vi "ScanDelay_FTIR_BBnorm_Aligning_NewportFlipper_AttenuateBB.vi"() -> ()   [LabVIEW 2022 SP3]
uses:
  Control_scanDelayWorkflow.ctl
  Control_GetSpectrum_BBnorm_AttenuateBB.ctl
panel:
  in  "Norm.smoothing":dbl=1.0 min=0.0 max=100.0 step=0.1
  in  "Flip anyway":bool
  out "Replicated wavelength (nm)":dbl
  in  "Piecewise flattening":i16 min=0 max=10 step=1
  in  "Sample atten.\npowers (%)":dbl[](array[numeric])=[100.0, 75.0, 50.0, 100.0, 100.0, 100.0]
  in  "Sample power (%)":dbl(slide)=100.0 min=0.0 max=100.0 scale=0.0..100.0
  in  "Cyc. per intfg. (BB)":i32=100
  out "Attenuation factor":dbl=1.0
  out "Replication wavelengths":dbl[](array[numeric])=[15000.0, 15000.0, 15000.0, 15000.0, 15000.0, 15000.0, 14286.0, 14286.0, 13333.0, 13333.0, 12500.0, 11765.0, 11111.0, 10526.0, 10000.0, 9524.0, 9091.0, 8696.0, 8333.0, 8000.0, 7692.0, 7407.0, 7143.0, 6897.0, 6667.0, 6452.0, 6250.0, 6061.0, 5882.0, 5714.0, 5556.0, 5405.0, 5263.0, 0.0]
  out "Replicator wavelengths loaded":bool=TRUE
  in  "Replic. path":path=path "C:/Users/mnopl/Desktop/Software/mnOPSuite/PRISM/Alpha replicator tables/2022.10.12_550-2000cm-1_ExtraExtraLowEnergy.txt"
  in  "Load replic. table":bool
  in  "BB attenuation\npowers (%)":dbl[](array[numeric])=[50.0, 1.5, 1.0, 2.0, 2.0, 2.0]
  in  "Attenuation\nenergies (cm-1)":dbl[](array[numeric])=[600.0, 1000.0, 1200.0, 1550.0, 1650.0, 1800.0]
  in  "BB power (%)":dbl(slide)=2.0202020202020203 min=0.0 max=100.0 scale=0.0..100.0
  in  "Power threshold":dbl(slide)=112.33240329780287 scale=10.0..1000.0
  in  "Update alignment":bool
  in  "Bright beam: alignment delay":i32=-11
  in  "Norm phase offset":dbl=14.7
  in  "Bright beam: physical channels (inputV, ScanDelay X)":tag="Dev1/ai2,Dev1/ai3"
  in  "Sample: physical channels (inputV, ScanDelay X)":tag="Dev1/ai6,Dev1/ai3"
  in  "Sample: alignment delay":i32=-2
  in  "Path to save\nnormalized spectrum":path=path "D:/Dropbox/Data/Park-SNOM/2022.10.24 - Alex undeformed STO/STO(Undeformed,S3)-to-Au(S3 x0.25).txt"
  in  "Save normalized\nspectrum":bool
  in  "Optimize\ninterferogram\nalignment":bool
  in  "Toggle BB\nmirror\nUp / Down":bool
  in  "Realign phase":bool=TRUE
  in  "Window FFT":bool=TRUE
  in  "Pause\nacquisition":bool
  in  "Replicate\nfrom #":i8 min=0
  in  "Envelope width":dbl(slide)=2.0303030303030303 scale=0.25..4.0
  out "Accumulated sample BB spectrum":dbl[][](array[numeric])=[[501.8020561554538, 506.7137372169034, 511.62541827835304, 516.5370993398027, 521.4487804012523, 526.3604614627019, 531.2721425241515, 536.1838235856012, 541.0955046470508, 546.0071857085004, 550.91886676995, 555.8305478313996, 560.7422288928493, 565.6539099542989, 570.5655910157485, 575.4772720771981, 580.3889531386478, 585.3006342000974, 590.212315261547, 595.1239963229966, 600.0356773844462, 604.9473584458959, 609.8590395073455, 614.7707205687951, 619.6824016302447, 624.5940826916944, 629.505763753144, 634.4174448145936, 639.3291258760432, 644.2408069374928, 649.1524879989424, 654.0641690603921, 658.9758501218417, 663.8875311832913, 668.799212244741, 673.7108933061907, 678.6225743676403, 683.5342554290899, 688.4459364905395, 693.357617551989, 698.2692986134388, 703.1809796748884, 708.092660736338, 713.0043417977877, 717.9160228592373, 722.8277039206869, 727.7393849821365, 732.6510660435861, 737.5627471050357, 742.4744281664854, 747.386109227935, 752.2977902893846, 757.2094713508343, 762.1211524122839, 767.0328334737335, 771.9445145351831, 776.8561955966327, 781.7678766580823, 786.6795577195319, 791.5912387809816, 796.5029198424312, 801.4146009038809, 806.3262819653305, 811.2379630267801, 816.1496440882297, 821.0613251496793, 825.9730062111289, 830.8846872725785, 835.7963683340282, 840.7080493954778, 845.6197304569275, 850.5314115183771, 855.4430925798267, 860.3547736412763, 865.2664547027259, 870.1781357641755, 875.0898168256251, 880.0014978870748, 884.9131789485244, 889.8248600099741, 894.7365410714237, 899.6482221328733, 904.5599031943229, 909.4715842557725, 914.3832653172221, 919.2949463786717, 924.2066274401215, 929.118308501571, 934.0299895630206, 938.9416706244704, 943.85335168592, 948.7650327473696, 953.6767138088192, 958.5883948702688, 963.5000759317184, 968.4117569931681, 973.3234380546177, 978.2351191160673, 983.146800177517, 988.0584812389666, 992.9701623004162, 997.8818433618658, 1002.7935244233154, 1007.705205484765, 1012.6168865462147, 1017.5285676076643, 1022.4402486691139, 1027.3519297305634, 1032.2636107920132, 1037.1752918534628, 1042.0869729149124, 1046.998653976362, 1051.9103350378116, 1056.8220160992614, 1061.733697160711, 1066.6453782221606, 1071.5570592836102, 1076.4687403450598, 1081.3804214065094, 1086.292102467959, 1091.2037835294086, 1096.1154645908582, 1101.0271456523078, 1105.9388267137574, 1110.850507775207, 1115.7621888366566, 1120.6738698981064, 1125.585550959556, 1130.4972320210056, 1135.4089130824552, 1140.3205941439048, 1145.2322752053547, 1150.1439562668043, 1155.0556373282539, 1159.9673183897035, 1164.878999451153, 1169.7906805126026, 1174.7023615740522, 1179.6140426355018, 1184.5257236969514, 1189.437404758401, 1194.3490858198506, 1199.2607668813002, 1204.1724479427498, 1209.0841290041997, 1213.9958100656493, 1218.9074911270989, 1223.8191721885485, 1228.730853249998, 1233.642534311448, 1238.5542153728975, 1243.465896434347, 1248.3775774957967, 1253.2892585572463, 1258.2009396186959, 1263.1126206801455, 1268.024301741595, 1272.9359828030447, 1277.8476638644943, 1282.7593449259439, 1287.6710259873935, 1292.582707048843, 1297.4943881102927, 1302.4060691717425, 1307.317750233192, 1312.2294312946417, 1317.1411123560913, 1322.0527934175411, 1326.9644744789907, 1331.8761555404403, 1336.78783660189, 1341.6995176633395, 1346.6111987247891, 1351.5228797862387, 1356.4345608476883, 1361.346241909138, 1366.2579229705875, 1371.1696040320371, 1376.0812850934867, 1380.9929661549363, 1385.904647216386, 1390.8163282778357, 1395.7280093392853, 1400.639690400735, 1405.5513714621845, 1410.4630525236341, 1415.374733585084, 1420.2864146465336, 1425.1980957079832, 1430.1097767694328, 1435.0214578308824, 1439.933138892332, 1444.8448199537816, 1449.7565010152312, 1454.6681820766808, 1459.5798631381303, 1464.49154419958, 1469.4032252610295, 1474.3149063224791, 1479.226587383929, 1484.1382684453786, 1489.0499495068282, 1493.9616305682778, 1498.8733116297274, 1503.7849926911772, 1508.6966737526268, 1513.6083548140764, 1518.520035875526, 1523.4317169369756, 1528.3433979984252, 1533.2550790598748, 1538.1667601213244, 1543.078441182774, 1547.9901222442236, 1552.9018033056732, 1557.813484367123, 1562.7251654285726, 1567.6368464900222, 1572.5485275514718, 1577.4602086129214, 1582.371889674371, 1587.2835707358206, 1592.1952517972702, 1597.1069328587198, 1602.0186139201694, 1606.9302949816192, 1611.8419760430688, 1616.7536571045184, 1621.665338165968, 1626.5770192274176, 1631.4887002888672, 1636.4003813503168, 1641.3120624117664, 1646.223743473216, 1651.1354245346658, 1656.0471055961154, 1660.958786657565, 1665.8704677190146, 1670.7821487804642, 1675.6938298419138, 1680.6055109033634, 1685.517191964813, 1690.4288730262626, 1695.3405540877125, 1700.252235149162, 1705.1639162106117, 1710.0755972720613, 1714.9872783335109, 1719.8989593949605, 1724.81064045641, 1729.7223215178597, 1734.6340025793093, 1739.545683640759, 1744.4573647022087, 1749.3690457636583, 1754.2807268251079, 1759.1924078865575, 1764.104088948007, 1769.0157700094567, 1773.9274510709063, 1778.8391321323559, 1783.7508131938057, 1788.6624942552553, 1793.574175316705, 1798.4858563781545, 1803.397537439604, 1808.3092185010537, 1813.2208995625033, 1818.132580623953, 1823.0442616854025, 1827.9559427468523, 1832.867623808302, 1837.7793048697515, 1842.690985931201, 1847.6026669926507, 1852.5143480541003, 1857.42602911555, 1862.3377101769995, 1867.249391238449, 1872.161072299899, 1877.0727533613485, 1881.9844344227981, 1886.8961154842477, 1891.8077965456973, 1896.719477607147, 1901.6311586685965, 1906.5428397300461, 1911.4545207914957, 1916.3662018529456, 1921.2778829143951, 1926.1895639758447, 1931.1012450372943, 1936.012926098744, 1940.9246071601935, 1945.8362882216431, 1950.7479692830927, 1955.6596503445423, 1960.571331405992, 1965.4830124674418, 1970.3946935288914, 1975.306374590341, 1980.2180556517906, 1985.1297367132402, 1990.0414177746898, 1994.9530988361394, 1999.864779897589], [9.05414272477129e-06, 1.146072070056428e-05, 1.3531434917469873e-05, 1.5257339061957748e-05, 1.7079437144261535e-05, 1.8586424060074166e-05, 1.9304052743786562e-05, 1.999383336317147e-05, 2.1561334770228305e-05, 2.2279284302473234e-05, 2.2799783386304058e-05, 2.3335960682250692e-05, 2.3711409589322383e-05, 2.3012041962517163e-05, 2.092371318189444e-05, 1.8247728538339973e-05, 1.6369451359050923e-05, 1.8071206366236603e-05, 2.2128161852382288e-05, 2.6588390553069066e-05, 3.040115189109792e-05, 3.4074633486252515e-05, 3.663854308845291e-05, 3.8686950213374986e-05, 3.998630059395697e-05, 4.036558448352778e-05, 3.9767897466925815e-05, 3.83635045958129e-05, 3.879241420070519e-05, 4.375572948539814e-05, 4.860211083641365e-05, 5.239661368228191e-05, 5.381305658605131e-05, 5.4605335585803846e-05, 5.456928023046857e-05, 5.330826922593081e-05, 5.155650135346775e-05, 4.963808606724598e-05, 4.7300273768685975e-05, 4.4789283821985914e-05, 4.172821833381964e-05, 3.8522819240302246e-05, 3.534413510043003e-05, 3.109825854574018e-05, 2.789151288182236e-05, 2.477637717894916e-05, 2.1665916765090898e-05, 1.8094472804190557e-05, 1.3885132135543352e-05, 1.3855836966766698e-05, 1.9174946576800012e-05, 2.288883487652522e-05, 2.736044057404942e-05, 3.2660182184323965e-05, 3.805551290684421e-05, 4.1634230858486924e-05, 4.359515344804649e-05, 4.417192112484465e-05, 4.350418637820082e-05, 4.159838227870174e-05, 3.863530651558005e-05, 3.689047831293406e-05, 3.564065659373262e-05, 3.4741453422092514e-05, 3.491100256574226e-05, 3.562501222570058e-05, 3.815400212911604e-05, 4.088615936631992e-05, 4.4000391910526505e-05, 4.695543922507996e-05, 4.8434044740882187e-05, 5.061622452333294e-05, 5.4756769204182285e-05, 5.758236758016324e-05, 5.669735052184797e-05, 5.42170352495056e-05, 5.308083060926907e-05, 4.804897607315596e-05, 4.092594837741294e-05, 3.717690682741493e-05, 3.743689734221249e-05, 4.026107820119904e-05, 4.4954407209320324e-05, 4.7937791250041886e-05, 5.0697804141281584e-05, 5.409179272902676e-05, 5.5051425613154196e-05, 5.943098268745728e-05, 6.02792792414743e-05, 6.196699298401036e-05, 6.397471069494848e-05, 6.66199487409774e-05, 7.127680886195002e-05, 7.458691093424846e-05, 7.731337733913675e-05, 7.785117839195202e-05, 7.53822505861062e-05, 7.056970040413338e-05, 6.291131100671327e-05, 5.2941329091929496e-05, 4.392391802194871e-05, 3.963449945856646e-05, 4.1953719475290424e-05, 4.771653614820673e-05, 5.335544843090435e-05, 5.616090792749654e-05, 5.562053151302489e-05, 5.21377627896389e-05, 4.501523397633283e-05, 3.249677831618434e-05, 1.7141861274259747e-05, 1.5912097509484014e-05, 3.462175484396277e-05, 5.7583346557761405e-05, 7.888606886101375e-05, 9.918158620308137e-05, 0.0001155235452915555, 0.0001289014913062019, 0.00013971733824365195, 0.0001470980604228987, 0.00015492802482606013, 0.00016264966498361625, 0.00016940708362537147, 0.00017497322968332827, 0.00018102746470570247, 0.0001870200933101339, 0.0001903175596330271, 0.00018897095803169608, 0.00018550126083230982, 0.00017557385544742657, 0.0001607038012571914, 0.0001367544362581611, 0.00010578345348198371, 8.546921892384217e-05, 9.52720614452018e-05, 0.00013011849973922022, 0.00019168098489810164, 0.00026725317849966666, 0.0003465746427620213, 0.00042891126018012405, 0.0005125761092231905, 0.0006132560660052971, 0.0007934024917234689, 0.001148817600728305, 0.0017821667597155177, 0.002718769896826103, 0.004011495255399954, 0.005669136912491277, 0.0076513168713931235, 0.009982636477995343, 0.012501134269760187, 0.015024090173468677, 0.017527550291906425, 0.019536079280951586, 0.020963553367104662, 0.021737970184997124, 0.021567120315550893, 0.020651465456608627, 0.019327507634875202, 0.017587385259346063, 0.015027071922176814, 0.01172814204759582, 0.008774676653795286, 0.0058183670585716905, 0.003766850285673133, 0.002212783419764623, 0.0012805222286522478, 0.0009088416748197714, 0.0008030169245465611, 0.0007363552520419021, 0.0006601492505867679, 0.0005736996220301791, 0.00046609251899519294, 0.0003437566881312927, 0.00022903562440392688, 0.00012838136651867715, 6.056117939395001e-05, 5.030059625889761e-05, 9.37824759573024e-05, 0.0001365567600822889, 0.00017761940643246386, 0.00020480688388601666, 0.0002213234600721696, 0.00023091740660175332, 0.00023050029871893855, 0.00022282558171466467, 0.00021176685424416765, 0.00020022832886297797, 0.0001912226868460405, 0.00018495657878795033, 0.00017852095629343115, 0.0001715729510544182, 0.0001653927454598181, 0.00015813440587111882, 0.00014740866431915028, 0.00013075370521333123, 0.00011249410778699135, 9.14522961639837e-05, 7.030504947509215e-05, 4.8274400107189045e-05, 3.182127229372215e-05, 2.4193419332374132e-05, 2.7592839368661025e-05, 3.8138419024464994e-05, 4.7411364923720376e-05, 5.453880382281337e-05, 5.900190986884964e-05, 5.939162416780368e-05, 5.836904180156344e-05, 5.7601729757341124e-05, 5.995501366208591e-05, 6.650413636839761e-05, 7.791655511014081e-05, 9.023797696062717e-05, 0.0001015790770096666, 0.00010948200015457708, 0.00011526639888839689, 0.00011795109028559512, 0.00011608954265675919, 0.00011154380593283861, 0.0001044640218107466, 9.618589325302785e-05, 8.897245175579604e-05, 8.297362182561573e-05, 7.733197817718043e-05, 7.221453820714107e-05, 6.798010472825792e-05, 6.209106017009621e-05, 5.582616105465967e-05, 4.889814882305325e-05, 4.308432303836618e-05, 3.81468507684591e-05, 3.504836304277521e-05, 3.3606430234370614e-05, 3.4892670864467355e-05, 3.740416873433292e-05, 4.014239344052927e-05, 4.236918893226478e-05, 4.540812717648292e-05, 4.750654552892193e-05, 4.88451465477639e-05, 4.999628837926609e-05, 5.0693745130209864e-05, 4.965733153995291e-05, 4.7718157132532524e-05, 4.47814947400894e-05, 4.222961881813198e-05, 4.363887345181102e-05, 4.4957856221667463e-05, 4.51818357062012e-05, 4.386171390158789e-05, 4.201732174854946e-05, 4.069355966749328e-05, 4.057027674774872e-05, 3.956998660491812e-05, 3.7473432147203064e-05, 3.470264995956467e-05, 3.080829371952867e-05, 2.5482362826008645e-05, 1.9424338594941943e-05, 1.5159327710234029e-05, 1.2079206222871872e-05, 1.0651298178296682e-05, 1.2330602779842834e-05, 1.4976309843244352e-05, 1.677832393183783e-05, 1.7707514496502166e-05, 1.8518224272784254e-05, 2.0645123455280968e-05, 2.238958039060859e-05, 2.4439615813823628e-05, 2.6411783669056102e-05, 2.9293749268361072e-05, 3.226870700779618e-05, 3.5575707796609386e-05, 3.8953809781552114e-05, 4.235176618092753e-05, 4.514116087133663e-05, 4.6540114190942e-05, 4.606769214915828e-05, 4.491425812718059e-05, 4.383267184081204e-05, 4.511594164863621e-05, 4.841621611549014e-05, 5.084628744927319e-05, 5.1740258164234994e-05, 5.180678588447729e-05, 5.1365569739836615e-05, 5.05500855713967e-05, 4.8324346627633626e-05, 4.368426081651136e-05, 3.9215637554996545e-05, 3.559618337661666e-05, 3.2627452977102426e-05, 2.9761293070238496e-05, 2.7353219897512085e-05, 2.533622978939261e-05, 2.3270055938289895e-05, 2.161392330779274e-05, 2.0154870308401806e-05, 1.9462572929597903e-05, 2.0037053102543743e-05, 2.121962262822815e-05, 2.207763674218256e-05, 2.318570856142014e-05, 2.352550308647713e-05], [0.6806744259585175, 0.6849882092343899, 0.668495848466184, 0.613823660290151, 0.5670256699905454, 0.5445875440523031, 0.546990064137304, 0.5027971094006224, 0.47163747526178623, 0.48842909948987007, 0.5171189634151799, 0.4957475740429013, 0.4888192862937894, 0.4922446845138241, 0.4830547740167819, 0.4523330038331212, 0.43934481192281666, 0.41091648448910995, 0.3701383178282937, 0.2576704200895707, -0.05406794808844366, -2.9309765509939187, -2.9831352822886825, -3.0198247651169337, -3.0713371549259603, -3.114948189689566, -3.1491367580851777, -3.1451705410699007, -3.129289925753888, -3.125575394129504, -3.106096390749937, -3.100847728135735, -3.135358025017434, -3.1838151253039304, -3.2648924033810016, -3.376909723106753, -3.541691857634501, -3.7798495395501477, -4.02201586442248, -4.195031710908829, -4.347412820078549, -4.456887451307068, -4.546803544906954, -4.635519524113365, -4.66545309054276, -4.68530639093207, -4.691936585983891, -4.708317262997989, -4.544956516040903, -4.084744355381776, -3.5889760371687154, -3.236601839820825, -2.9726808507353693, -2.800779807057664, -2.7200603857023293, -2.645324467735087, -2.5994992809400856, -2.5712444774069074, -2.5101737131124016, -2.3835934415958673, -2.2020112502296567, -1.848566034791038, -1.539120582293457, -1.2876672100153965, -1.1712491575884099, -1.1983291631701047, -1.2457471069620216, -1.3567799632556796, -1.4782346677529863, -1.5469386689494908, -1.6102464660586944, -1.6331750864817036, -1.6709023484297494, -1.6881838117255588, -1.5945841111901449, -1.4564987015925728, -1.3313807472150505, -1.021834509760915, -0.6265802400027387, -0.3933956777218133, -0.23455529944051934, -0.116393575522356, -0.06063583465495674, -0.056672229363642176, -0.0707011853554041, -0.06651556862565093, -0.06701995189815028, -0.08519836384250516, -0.1453752673935758, -0.19104373919919887, -0.24310016886619273, -0.2731146058472622, -0.29908174145078853, -0.3459180439848564, -0.38095926307008954, -0.4168769040451293, -0.4411278698630139, -0.4798539476175496, -0.5449944482579601, -0.6581009327727547, -0.8715676027976937, -1.2508736277829517, -1.6971337421250543, -2.0213691446290594, -2.2040449228837145, -2.266631075624979, -2.2641540356125422, -2.2365377454531417, -2.1599287851486655, -2.0463023119591957, -1.6165662075490066, -0.41549872588223785, 0.21706889676303426, 0.34458978885153213, 0.36340627078730087, 0.36919498924122207, 0.3524838424701317, 0.3204822645118805, 0.2957596233332462, 0.28578266456548057, 0.2848106483127703, 0.29956801355058665, 0.3209924016384131, 0.35097351985282144, 0.3893186436017326, 0.423902712704169, 0.44627800290509206, 0.46298635487752854, 0.47871335326365333, 0.4905963210656376, 0.4841124897370323, 0.45541657032287786, 0.3652951332237495, 0.04303936858528297, -0.7536743878984394, -1.3261829974428108, -1.4696028844701314, -1.4586429486007302, -1.3840109453291167, -1.2516588040654963, -1.0573123759968088, -0.7824538427101194, -0.4474818694363703, -0.13589815712052247, 0.08755263607200398, 0.21642632980081397, 0.2862942277725255, 0.3205893750742272, 0.3326444570982469, 0.32938127045895227, 0.31833349636619657, 0.30329049194792596, 0.2829553232250954, 0.26687390368277114, 0.2555619318755968, 0.2505673029245083, 0.25911595629275597, 0.2772754960838983, 0.2973425409459973, 0.3029649582927613, 0.2827761405262055, 0.23732942507677943, 0.20163466037668648, 0.1331497607854461, 0.0379820195901774, -0.13999981345004334, -0.47795745571318854, -0.929010937914907, -1.1994103072581521, -1.2896615783323253, -1.2653352298683456, -1.2098483095719286, -1.1657699548059104, -1.1471930383624103, -1.1281429911558267, -1.1795391975895133, -1.5039067718021788, -2.6936269684786187, -3.0664592616953006, -3.1193851903000795, -3.0854087414640223, -3.0549441336742693, -3.0184550566806156, -2.985441049200191, -2.9511412813394178, -2.918187087297462, -2.8907032121741385, -2.854900914838226, -2.834920748588893, -2.8245153356991257, -2.819751606455825, -2.81602192316084, -2.8152291411993464, -2.829577389185467, -2.8550562214387445, -2.8903925112420272, -2.9264918455310682, -2.9616994840566666, -3.0002506084331704, -2.999118248425433, -2.845589508335458, -1.7373949316942547, -0.6932921798700211, -0.5384382613525608, -0.4995766927485695, -0.514316046620444, -0.5745218661614621, -0.669775445573983, -0.8239144445259048, -1.0346387042374663, -1.2990121854938654, -1.5986247869854187, -1.8472296623316287, -2.021497282413414, -2.1466514781422963, -2.209378153096481, -2.2424589750897685, -2.266648851082515, -2.2799797005398905, -2.309912237678326, -2.345692915641117, -2.384757375923997, -2.4363018382807486, -2.497667099925217, -2.564332792856057, -2.6256948434904293, -2.6694663154440907, -2.6932662176610767, -2.671755748082959, -2.6121329426752458, -2.50396224079028, -2.405377043888912, -2.261188670924277, -1.961869475625591, -1.5078157042629958, -1.0919329006878589, -0.9008797089504061, -0.7780224728162258, -0.7243893273929989, -0.7048124869470134, -0.7013557014828184, -0.7108512635927231, -0.7253035863197828, -0.75849837833151, -0.8028701121530308, -0.8536743084239977, -0.8917074118238381, -0.9071203609288722, -0.9242697845010359, -0.9038786131617589, -0.8639937766237017, -0.8339523553539512, -0.7597506511491052, -0.6887229433663866, -0.6537523468968877, -0.6544456961542199, -0.6418528873431063, -0.6508048799553668, -0.7173890701039488, -0.8823720275302099, -1.234560542288769, -2.5487899960284257, -3.265859158892774, -3.4350535154588333, -3.5483551781026894, -3.613569542051124, -3.7209267603498977, -3.8838812245739764, -4.105786402002394, -4.4040108873667805, -4.694065779254025, -4.93405521235141, -5.132177325063402, -5.324967330883069, -5.4728872622221445, -5.590032554039752, -5.677328649274422, -5.752216276239508, -5.805457545657504, -5.843483612071168, -5.869153092716736, -5.920157198340206, -5.959502513483272, -6.0264303723496795, -6.140367982249792, -6.326400049319197, -6.6048321771131455, -7.029094864507549, -7.572319323971797, -8.001401477157643, -8.185674079242062, -8.311840842830115, -8.424449363726211, -8.502254435462461, -8.533576338364043, -8.580247369363327, -8.583386316082233, -8.587663480138602, -8.609199879121022, -8.632127356897414, -8.59206944725306, -8.502866290557257, -8.413064474235739, -8.331740024107319, -8.268889123446257, -8.255981731146719]]
  out "Accumulated sample spectrum":dbl[][](array[numeric])=[[501.8020561554538, 506.7137372169034, 511.62541827835304, 516.5370993398027, 521.4487804012523, 526.3604614627019, 531.2721425241515, 536.1838235856012, 541.0955046470508, 546.0071857085004, 550.91886676995, 555.8305478313996, 560.7422288928493, 565.6539099542989, 570.5655910157485, 575.4772720771981, 580.3889531386478, 585.3006342000974, 590.212315261547, 595.1239963229966, 600.0356773844462, 604.9473584458959, 609.8590395073455, 614.7707205687951, 619.6824016302447, 624.5940826916944, 629.505763753144, 634.4174448145936, 639.3291258760432, 644.2408069374928, 649.1524879989424, 654.0641690603921, 658.9758501218417, 663.8875311832913, 668.799212244741, 673.7108933061907, 678.6225743676403, 683.5342554290899, 688.4459364905395, 693.357617551989, 698.2692986134388, 703.1809796748884, 708.092660736338, 713.0043417977877, 717.9160228592373, 722.8277039206869, 727.7393849821365, 732.6510660435861, 737.5627471050357, 742.4744281664854, 747.386109227935, 752.2977902893846, 757.2094713508343, 762.1211524122839, 767.0328334737335, 771.9445145351831, 776.8561955966327, 781.7678766580823, 786.6795577195319, 791.5912387809816, 796.5029198424312, 801.4146009038809, 806.3262819653305, 811.2379630267801, 816.1496440882297, 821.0613251496793, 825.9730062111289, 830.8846872725785, 835.7963683340282, 840.7080493954778, 845.6197304569275, 850.5314115183771, 855.4430925798267, 860.3547736412763, 865.2664547027259, 870.1781357641755, 875.0898168256251, 880.0014978870748, 884.9131789485244, 889.8248600099741, 894.7365410714237, 899.6482221328733, 904.5599031943229, 909.4715842557725, 914.3832653172221, 919.2949463786717, 924.2066274401215, 929.118308501571, 934.0299895630206, 938.9416706244704, 943.85335168592, 948.7650327473696, 953.6767138088192, 958.5883948702688, 963.5000759317184, 968.4117569931681, 973.3234380546177, 978.2351191160673, 983.146800177517, 988.0584812389666, 992.9701623004162, 997.8818433618658, 1002.7935244233154, 1007.705205484765, 1012.6168865462147, 1017.5285676076643, 1022.4402486691139, 1027.3519297305634, 1032.2636107920132, 1037.1752918534628, 1042.0869729149124, 1046.998653976362, 1051.9103350378116, 1056.8220160992614, 1061.733697160711, 1066.6453782221606, 1071.5570592836102, 1076.4687403450598, 1081.3804214065094, 1086.292102467959, 1091.2037835294086, 1096.1154645908582, 1101.0271456523078, 1105.9388267137574, 1110.850507775207, 1115.7621888366566, 1120.6738698981064, 1125.585550959556, 1130.4972320210056, 1135.4089130824552, 1140.3205941439048, 1145.2322752053547, 1150.1439562668043, 1155.0556373282539, 1159.9673183897035, 1164.878999451153, 1169.7906805126026, 1174.7023615740522, 1179.6140426355018, 1184.5257236969514, 1189.437404758401, 1194.3490858198506, 1199.2607668813002, 1204.1724479427498, 1209.0841290041997, 1213.9958100656493, 1218.9074911270989, 1223.8191721885485, 1228.730853249998, 1233.642534311448, 1238.5542153728975, 1243.465896434347, 1248.3775774957967, 1253.2892585572463, 1258.2009396186959, 1263.1126206801455, 1268.024301741595, 1272.9359828030447, 1277.8476638644943, 1282.7593449259439, 1287.6710259873935, 1292.582707048843, 1297.4943881102927, 1302.4060691717425, 1307.317750233192, 1312.2294312946417, 1317.1411123560913, 1322.0527934175411, 1326.9644744789907, 1331.8761555404403, 1336.78783660189, 1341.6995176633395, 1346.6111987247891, 1351.5228797862387, 1356.4345608476883, 1361.346241909138, 1366.2579229705875, 1371.1696040320371, 1376.0812850934867, 1380.9929661549363, 1385.904647216386, 1390.8163282778357, 1395.7280093392853, 1400.639690400735, 1405.5513714621845, 1410.4630525236341, 1415.374733585084, 1420.2864146465336, 1425.1980957079832, 1430.1097767694328, 1435.0214578308824, 1439.933138892332, 1444.8448199537816, 1449.7565010152312, 1454.6681820766808, 1459.5798631381303, 1464.49154419958, 1469.4032252610295, 1474.3149063224791, 1479.226587383929, 1484.1382684453786, 1489.0499495068282, 1493.9616305682778, 1498.8733116297274, 1503.7849926911772, 1508.6966737526268, 1513.6083548140764, 1518.520035875526, 1523.4317169369756, 1528.3433979984252, 1533.2550790598748, 1538.1667601213244, 1543.078441182774, 1547.9901222442236, 1552.9018033056732, 1557.813484367123, 1562.7251654285726, 1567.6368464900222, 1572.5485275514718, 1577.4602086129214, 1582.371889674371, 1587.2835707358206, 1592.1952517972702, 1597.1069328587198, 1602.0186139201694, 1606.9302949816192, 1611.8419760430688, 1616.7536571045184, 1621.665338165968, 1626.5770192274176, 1631.4887002888672, 1636.4003813503168, 1641.3120624117664, 1646.223743473216, 1651.1354245346658, 1656.0471055961154, 1660.958786657565, 1665.8704677190146, 1670.7821487804642, 1675.6938298419138, 1680.6055109033634, 1685.517191964813, 1690.4288730262626, 1695.3405540877125, 1700.252235149162, 1705.1639162106117, 1710.0755972720613, 1714.9872783335109, 1719.8989593949605, 1724.81064045641, 1729.7223215178597, 1734.6340025793093, 1739.545683640759, 1744.4573647022087, 1749.3690457636583, 1754.2807268251079, 1759.1924078865575, 1764.104088948007, 1769.0157700094567, 1773.9274510709063, 1778.8391321323559, 1783.7508131938057, 1788.6624942552553, 1793.574175316705, 1798.4858563781545, 1803.397537439604, 1808.3092185010537, 1813.2208995625033, 1818.132580623953, 1823.0442616854025, 1827.9559427468523, 1832.867623808302, 1837.7793048697515, 1842.690985931201, 1847.6026669926507, 1852.5143480541003, 1857.42602911555, 1862.3377101769995, 1867.249391238449, 1872.161072299899, 1877.0727533613485, 1881.9844344227981, 1886.8961154842477, 1891.8077965456973, 1896.719477607147, 1901.6311586685965, 1906.5428397300461, 1911.4545207914957, 1916.3662018529456, 1921.2778829143951, 1926.1895639758447, 1931.1012450372943, 1936.012926098744, 1940.9246071601935, 1945.8362882216431, 1950.7479692830927, 1955.6596503445423, 1960.571331405992, 1965.4830124674418, 1970.3946935288914, 1975.306374590341, 1980.2180556517906, 1985.1297367132402, 1990.0414177746898, 1994.9530988361394, 1999.864779897589], [7.096082360479396e-06, 1.6220386856729275e-05, 1.2223386866077108e-05, 4.282334903322743e-06, 2.1097332179997113e-05, 1.5931965038395668e-05, 1.4783115049740189e-05, 1.064874887303893e-05, 1.5448597881790268e-05, 1.3470240412791832e-05, 1.2958578997869333e-05, 1.5342759416644122e-05, 3.0360154405360435e-06, 7.328117975916059e-06, 1.11069522683048e-05, 1.348424065152223e-05, 1.5966667764614643e-05, 4.256482081007854e-06, 7.698741492917485e-06, 8.865391382740525e-06, 1.8176244058347554e-05, 1.8973154162308674e-05, 1.0912895095445991e-05, 1.325424212557706e-05, 1.084767493023024e-05, 8.18491392927694e-06, 1.0172923454735038e-05, 8.606235895685828e-06, 7.1929677374480615e-06, 6.208684786759582e-06, 1.3033603740988862e-05, 1.729592544754774e-05, 1.1632791731803707e-05, 6.270479610479669e-06, 1.9015952315639412e-05, 1.5877692037602524e-05, 1.424704035985526e-05, 1.3417783494287481e-05, 4.9624588871503026e-06, 7.920464022574053e-06, 7.754802113000556e-06, 1.2212327060122936e-05, 8.192239421572929e-06, 1.1878952892783207e-05, 7.2610520788568465e-06, 1.2441571480584719e-05, 7.0617603301759675e-06, 8.882572928968195e-06, 9.61627100927289e-06, 1.1613496964703238e-05, 1.2974020437570576e-05, 1.2539589787029214e-05, 1.3706075083989123e-05, 1.1166744177971556e-05, 1.09170847990934e-05, 1.396961345036368e-05, 6.148960410007418e-06, 4.117329979906626e-06, 8.251216270028971e-06, 1.4277654679068755e-05, 1.6989586466865932e-05, 9.830933833137905e-06, 2.5365020050501013e-06, 1.2505769826231134e-05, 9.948332249916361e-06, 2.022298421450121e-05, 2.2104870640054155e-05, 1.5351986693574494e-05, 1.6536808333752614e-05, 8.619346205853348e-06, 4.9269921873958635e-06, 7.539082415766658e-06, 1.1265265208212509e-05, 5.3093876408056685e-06, 1.8267496478440106e-05, 8.418129697236088e-06, 1.668977119652175e-05, 1.437691992133319e-05, 1.0733286491980835e-05, 8.030611362074507e-06, 5.290594276412685e-06, 8.325384417407644e-06, 9.164514378310757e-06, 9.132109210043603e-06, 8.92735511203776e-06, 8.642137938522881e-06, 8.43088721396767e-06, 1.5414142206645658e-05, 1.8917345530536863e-05, 1.6807294558207432e-05, 1.5562644438291655e-05, 2.191328348810439e-05, 1.562190993514149e-05, 2.35758717026132e-05, 1.9461969952376293e-05, 2.1239892281209746e-05, 2.551464670387115e-05, 2.121022896753515e-05, 3.1034869497750934e-05, 3.054262223968249e-05, 2.814065303153361e-05, 3.24239667768052e-05, 3.210108331623405e-05, 2.7097569118739543e-05, 1.9549287586006928e-05, 1.920471433777232e-05, 2.085211165385107e-05, 1.9778428616472202e-05, 1.899682396436571e-05, 2.2360867458495652e-05, 1.2903923483678998e-05, 9.716356015491789e-06, 1.1024458431202365e-05, 2.46070382438526e-05, 1.5794963754151342e-05, 2.1988195738978594e-05, 2.2493434485802777e-05, 2.274916971304642e-05, 1.9043714451361174e-05, 3.2455571822991444e-05, 3.9426946712707426e-05, 3.149836580550327e-05, 2.364862770413785e-05, 3.459382392234399e-05, 3.2561050961055636e-05, 2.9750840723544186e-05, 4.532134256484172e-05, 4.442650356547751e-05, 5.3030150646254015e-05, 5.777877288392492e-05, 5.936488175937551e-05, 5.690611765759707e-05, 7.136207722539052e-05, 8.684952921157855e-05, 9.607880565961691e-05, 0.00010397996424653021, 0.00011251166112605888, 0.00011842748610103626, 0.00013925700343623112, 0.00015837228854517795, 0.00018885798104664812, 0.0002357890120263042, 0.0003266366648277566, 0.0004648887026358305, 0.0006663324974086461, 0.0009375934492479617, 0.001289889201388835, 0.0017096453396765817, 0.002195358775923772, 0.002755687667586425, 0.0032971491483591315, 0.003808239568810946, 0.0043694670800612295, 0.004710317324253723, 0.0049607131589019665, 0.005073330983895903, 0.004967087237416828, 0.004769405674776652, 0.00436718318605272, 0.003898901118832271, 0.00326947860920914, 0.0024247164383817844, 0.0015537542497215198, 0.0009721965292059489, 0.0006385748499156821, 0.0003639037640460496, 0.00017783106662409116, 4.7234590752977354e-05, 5.348402396475515e-05, 7.932582168632317e-05, 0.00010868712870559444, 0.00012073088242670934, 0.0001268464298254565, 0.00010751739967993342, 9.802452444909778e-05, 9.109296479305137e-05, 7.798937791952395e-05, 6.4630360392463e-05, 5.1186347717194496e-05, 4.0165022761351634e-05, 4.020839021217865e-05, 3.352705190877265e-05, 3.659022537370472e-05, 3.6047183378015574e-05, 4.402664879467927e-05, 4.173403239711788e-05, 3.7094326533374566e-05, 3.394696617813053e-05, 4.367802757900978e-05, 3.2407369324367004e-05, 3.0888878509555866e-05, 1.796549087525518e-05, 1.6813720693790422e-05, 1.2809437299114951e-05, 1.5125920904250285e-05, 2.179655521601398e-05, 1.4294757256413644e-05, 2.2769359972224953e-05, 2.272077561802974e-05, 1.501029549552028e-05, 1.5224573132860858e-05, 1.1097189981791928e-05, 2.003415699578107e-05, 2.3507740890240143e-05, 1.930736487515885e-05, 3.205176877613794e-05, 3.086052880894781e-05, 3.3237639300179554e-05, 2.8189470341541665e-05, 3.111370999854575e-05, 2.6077334296632935e-05, 2.524932846695447e-05, 2.875277983849729e-05, 2.6310361342494755e-05, 1.87381490192934e-05, 1.861669662325644e-05, 1.7149505464031797e-05, 1.529861533541566e-05, 9.48608645730043e-06, 1.647272876786718e-05, 1.394451953490884e-05, 1.482969749153723e-05, 1.3216652858618266e-05, 7.882712972293426e-06, 6.864781536648055e-06, 4.847759809587256e-06, 5.223428548175379e-06, 8.39573915560291e-06, 8.126667526531172e-06, 7.058328123353561e-06, 7.461150127794082e-06, 8.86426238947459e-06, 1.0946980191083884e-05, 1.324259674572552e-05, 7.971177651892419e-06, 6.664935172352915e-06, 7.032122453049047e-06, 1.2270507074891597e-05, 7.013781342280346e-06, 1.611372777133013e-05, 1.951527239201233e-05, 1.3669726488652514e-05, 8.573566860325885e-06, 7.860704247845982e-06, 9.435319117366857e-06, 1.2611836193932327e-05, 1.126447375953876e-05, 6.02637982793345e-06, 1.545897546346109e-05, 9.287884220712906e-06, 1.1464108097064425e-05, 8.891965582088907e-06, 7.082816008008784e-06, 3.394680172403156e-06, 1.2984101675619772e-05, 1.4964963888138804e-05, 9.448127598473755e-06, 1.2011629818937472e-05, 1.283072967680753e-05, 1.2534603065023814e-05, 7.070989746489091e-06, 1.0179637281450386e-05, 1.0538069586795832e-05, 6.852441095224346e-06, 1.2104186559758078e-05, 1.2538628754685724e-05, 8.284175957360816e-06, 8.650858436875346e-06, 6.750854466426396e-06, 8.432146312558232e-06, 4.507974550206405e-06, 1.0949793060888158e-05, 5.95388678352254e-06, 6.307335969170798e-06, 4.074228192718652e-06, 4.8618155781926654e-06, 1.0512250410263202e-05, 9.499415448978633e-06, 6.276383121874037e-06, 8.169746448445238e-06, 1.2036117271404059e-05, 6.996683099276729e-06, 6.372316970241091e-06, 5.0453959969180045e-06, 6.421931102118251e-06, 1.4015419112640523e-05, 8.548924967471335e-06, 1.088449721112743e-05, 6.692844505840714e-06, 9.780322496321983e-06, 7.83291243722902e-06, 8.35343437412176e-06, 1.3834821163292688e-05, 1.0642471950111049e-05, 1.030219925131364e-05, 7.4303662725959695e-06, 9.261497345916458e-06, 1.0674127331454052e-05, 1.295346646167355e-05, 1.1722741477800632e-05, 8.763110544237398e-06, 1.1406670493965474e-05, 1.2084041085027556e-05, 6.511018285955797e-06, 3.1419452991251818e-06, 6.047792812633947e-06], [-49.58206727087324, -52.06823293132049, -51.59677155767573, -52.31870069711781, -51.991164639108284, -51.05693027011136, -50.388390585021135, -50.67510232822931, -50.148745454930285, -53.19109093769427, -51.59616890898501, -49.96997724661843, -48.0637440852836, -46.17832069695589, -43.88779727601798, -44.54071428292487, -42.719929996739, -40.48253787695988, -38.13418935805937, -37.44789397470244, -36.369339805662136, -34.661575729363946, -32.53811809218756, -29.724037280654372, -27.318578053390738, -26.131113368174013, -25.79138634660744, -24.413830697153386, -24.532049098619993, -21.764139444463908, -19.768588590293476, -16.904423615168056, -15.570603067658666, -13.077056978181318, -11.922224489987983, -12.150316898367223, -10.859554185796085, -9.555622558304847, -7.624387873499771, -7.122390410818255, -7.266142534643009, -8.506066182506473, -6.762533961779596, -7.23859596712073, -8.583196058775755, -9.572516841189682, -8.231903811169232, -9.235464477024479, -9.316455438966969, -9.140920833410874, -9.165660825724288, -9.680412780771334, -9.394099306692553, -7.740358590358383, -7.804716406592078, -8.925910170046748, -7.57252877256316, -6.250146386562463, -8.288095994787668, -11.017446200235447, -9.175535888420548, -7.8714018716313845, -9.33669805879942, -9.349482128480396, -7.579829340238554, -10.48837944093927, -9.243334601881742, -10.27406749916372, -13.373102938096189, -11.771583040025796, -9.21987630645068, -10.457115391902867, -8.549877711788348, -5.588156527718432, -4.656552923516294, -4.352100257965269, -3.8128743676231167, -2.8369355809127157, -3.7777039410185225, -2.5078836341545454, -4.464358062030122, -5.47326755731185, -6.315870510377117, -9.023631774872982, -8.14176682870054, -5.648951000074462, -5.396575095619781, -2.7492283187998083, -0.9476749901979957, -1.6535079167293674, -1.9041012103507313, -1.4642522324003409, -1.5544175568067686, -1.5862247887869927, -1.4188927451235003, -1.3485365725741332, -1.4978984991802946, -1.6074631511796866, -1.1231856063554773, -0.9674954935016871, -0.9818292032517348, -1.4696951158149005, -1.3943436596178884, -1.2797707350272987, -1.0581472172672335, -1.2566924155893986, -0.8188802017241841, -0.934487379800018, -0.9201508576581574, -0.8364985504163798, -0.4854912152201365, -1.4813900102695783, -0.7551172904152708, -0.18569378918256518, 0.07691737929418707, -1.1067773466845523, -1.4570209687139908, -1.4317325333093294, -1.8580990895404312, -1.8836080909858168, -1.8368883765418644, -1.7590184052697708, -1.9554674043154279, -2.234847762600097, -1.7982446396746212, -2.2599299474556886, -2.1052395914099264, -2.022429445515499, -2.2702555833974003, -2.139098256382553, -2.400331377785264, -2.4125836446621207, -2.6703271276350478, -2.566581062856258, -2.7238206966689944, -2.7127621763842598, -2.7730758686688404, -2.9458740203269116, -2.897110094191291, -2.8571493576734355, -2.8373664847177764, -2.789842488116605, -2.7757876198668185, -2.7750969076867165, -2.730127253418047, -2.7416641966174637, -2.7615314886291316, -2.788149687873002, -2.8353974886299653, -2.865116417263593, -2.8976318239663357, -2.9525226237125963, -2.97852944270862, -3.0024743818616884, -3.031683030306553, -3.0314645913611997, -3.027047843178096, -2.9961596717096057, -2.9545397818372265, -2.93792034496191, -2.893638449305101, -2.8121468103189358, -2.9260995910297964, -2.963667938530378, -3.0741187876374028, -3.1249756345830946, -3.208674732285303, -3.597217737260891, -5.483519754354077, -5.849387636033342, -6.107262165211566, -6.140145056889352, -6.252678204666651, -6.250619717512635, -6.488896368472453, -6.44033235404315, -6.630118959397677, -6.635956163171599, -6.645818717841124, -6.528222838020028, -6.782348468449399, -6.708849169444861, -6.696444077887023, -6.746235629551208, -6.869028965930269, -6.861332623423706, -6.8207636106367175, -6.7994720656315195, -6.7998474237918884, -7.029169630898181, -6.992351732359666, -6.777250448594103, -7.012111012549369, -7.687826633074607, -7.437548686596088, -8.063193909697944, -8.340006034282496, -8.716808131153456, -8.439096372686564, -8.147286025639588, -6.9415702894675775, -8.045011049509114, -7.580931436108514, -7.278739704809638, -8.13649827499357, -7.772894666352457, -7.889164155367823, -7.827692780635076, -7.171712771117299, -7.296158022817778, -7.554901035468859, -7.7345530842275, -7.5111826383695615, -7.552248052429306, -7.550781763096708, -7.230642596223063, -7.447324426323249, -7.443610631135627, -7.439725797384867, -7.606296531013399, -7.785323317576015, -7.475011106511161, -6.98167908922936, -7.79089759710682, -6.726106551116871, -8.109015219159133, -7.462237261982594, -4.612723471222822, -3.7935231140733805, -5.216090924702357, -5.248598774188807, -4.15991094699082, -3.725230144267144, -6.858093955335086, -5.139396101609272, -5.360861136852755, -4.82214956875297, -3.753053779923313, -4.7960947914506065, -3.1275337418656264, -2.978161762441438, -2.8095698815112726, -4.079735670874875, -4.713059596127671, -1.7505931592448079, -3.8140547559468203, -3.5360568920327538, -2.2649426038786444, -0.04791412174990484, 0.6294052053287018, 0.1183832889078289, -0.548293474591425, 0.30766352864960567, -1.7009549342943515, -0.550868614347543, -0.387315192474297, -0.13119382138075508, -0.11547347909527872, -0.05089839595212453, -0.28486093981741334, 0.00043449825215446936, 1.0503147223107234, 0.15034553551333119, 1.5821608828076634, 1.899500705696532, -0.9754453882874543, -1.2905127638921385, -3.551211483864641, -6.297299968077951, -5.925915245102473, -8.303942056630753, -5.397154039382862, -8.31777800886968, -8.153461845292213, -5.929076766532205, -4.357415624658813, -1.9649943371332768, -0.6518423485552489, 0.35304915013031746, -2.1529003478899753, -0.2789829941474906, -0.8275960523606543, -1.5990956142781485, -1.2574528112380037, -1.1135107717981256, -1.0064545345404312, -0.6643235747175353, -2.1960638520043503, -1.4188220786783106, -1.68474878666958, -1.2845902439258552, -2.166556808127261, -1.962834740839405, -1.091371297982782, -0.9027447081329498, -1.963763228870782, -1.6989656292995718, -2.0681239676090044, -1.3241655749037804, -1.9706211964647977, -0.8286421870862952, -2.9765368288182827, -1.735695223359997, -0.9204437331073194, -2.2898437042328084, -1.840430591049298]]
  in  "BB-reference spectrum":bool
  in  "Acquire only\nBB 100% curve":bool
  in  "Toggle pause (ms)":dbl=4000.0
  out "BB-referenced spectrum (phase)":T1(graph)
  out "BB-referenced spectrum (amplitude)":T2(graph)
  out "Reference BB spectra":dbl[][](array[numeric])
  out "Reference spectra":dbl[][](array[numeric])
  out "Latest alpha cmd":string="@mir setpump 100.0"
  in  "Replicate\nalpha on\naccumulation":bool=TRUE
  out "# Accumulated":i32=2
  in  "Accumulate to #":i32=2
  in  "Cancel\nacquisition":bool
  out "Toggle position":i32=2
  out "Spectrum stored":bool=TRUE
  out "Reference stored":bool=TRUE
  out "Normalized spectrum (phase)":T1(graph)
  out "Normalized spectrum (amplitude)":T1(graph)
  in  "Store as reference":bool
  out "Python alpha rep path":path=path "C:/Users/mnopl/Desktop/software/mnOPSuite/PRISM/python/alpha.py"
  out "Activity status":string="Awaiting command"
  out "Acquisition status":string="Ready to acquire spectrum"
  in  "Path to save spectrum":path=path "D:/Dropbox/Data/Park-SNOM/2022.10.24 - Alex undeformed STO/Au(S3 x0.25).txt"
  in  "Load reference":bool
  in  "Path to load reference":path=path "D:/Dropbox/Data/Diagnostic/2022.11.02 - PRISM 100% lines/After colinearizing beam path/Au(4).txt"
  in  "Path to load spectrum":path=path "D:/Dropbox/Data/Diagnostic/2022.11.02 - PRISM 100% lines/After colinearizing beam path/Au(3).txt"
  in  "Apply spectral\nenvelope":bool=TRUE
  out "Binned interferogram":cluster{"X":dbl, "Y":dbl}[](graph)
  out "Sample BB Spectra":dbl[][](array[numeric])
  out "Sample Spectra":dbl[][](array[numeric])
  out "Python error: spectrum acquisition":errorcluster
  out "Python scandelay path":path=path "C:/Users/mnopl/Desktop/software/mnOPSuite/PRISM/python/scandelay_FTIR.py"
  in  "Time per\nacquisition (s)":dbl=0.18
  in  "Sampling rate":dbl=250000.0
  in  "Delay calibratior\nfactor (ps/V)":dbl=-2.38 format="%_6g"
  in  "Cyc. / intfg.\n(sample)":i32=100
  out "Accumulated spectrum (amplitude)":T3(graph)
  out "Acquisition cycle":dbl[][](graph)
  out "% averaged":dbl=100.0
  in  "Halt program":bool=TRUE
  out "Python error: activity loop":errorcluster
  in  "Load spectrum":bool
  in  "Save spectrum":bool
  in  "Normalize spectrum":bool
  in  "Acquire spectrum":bool
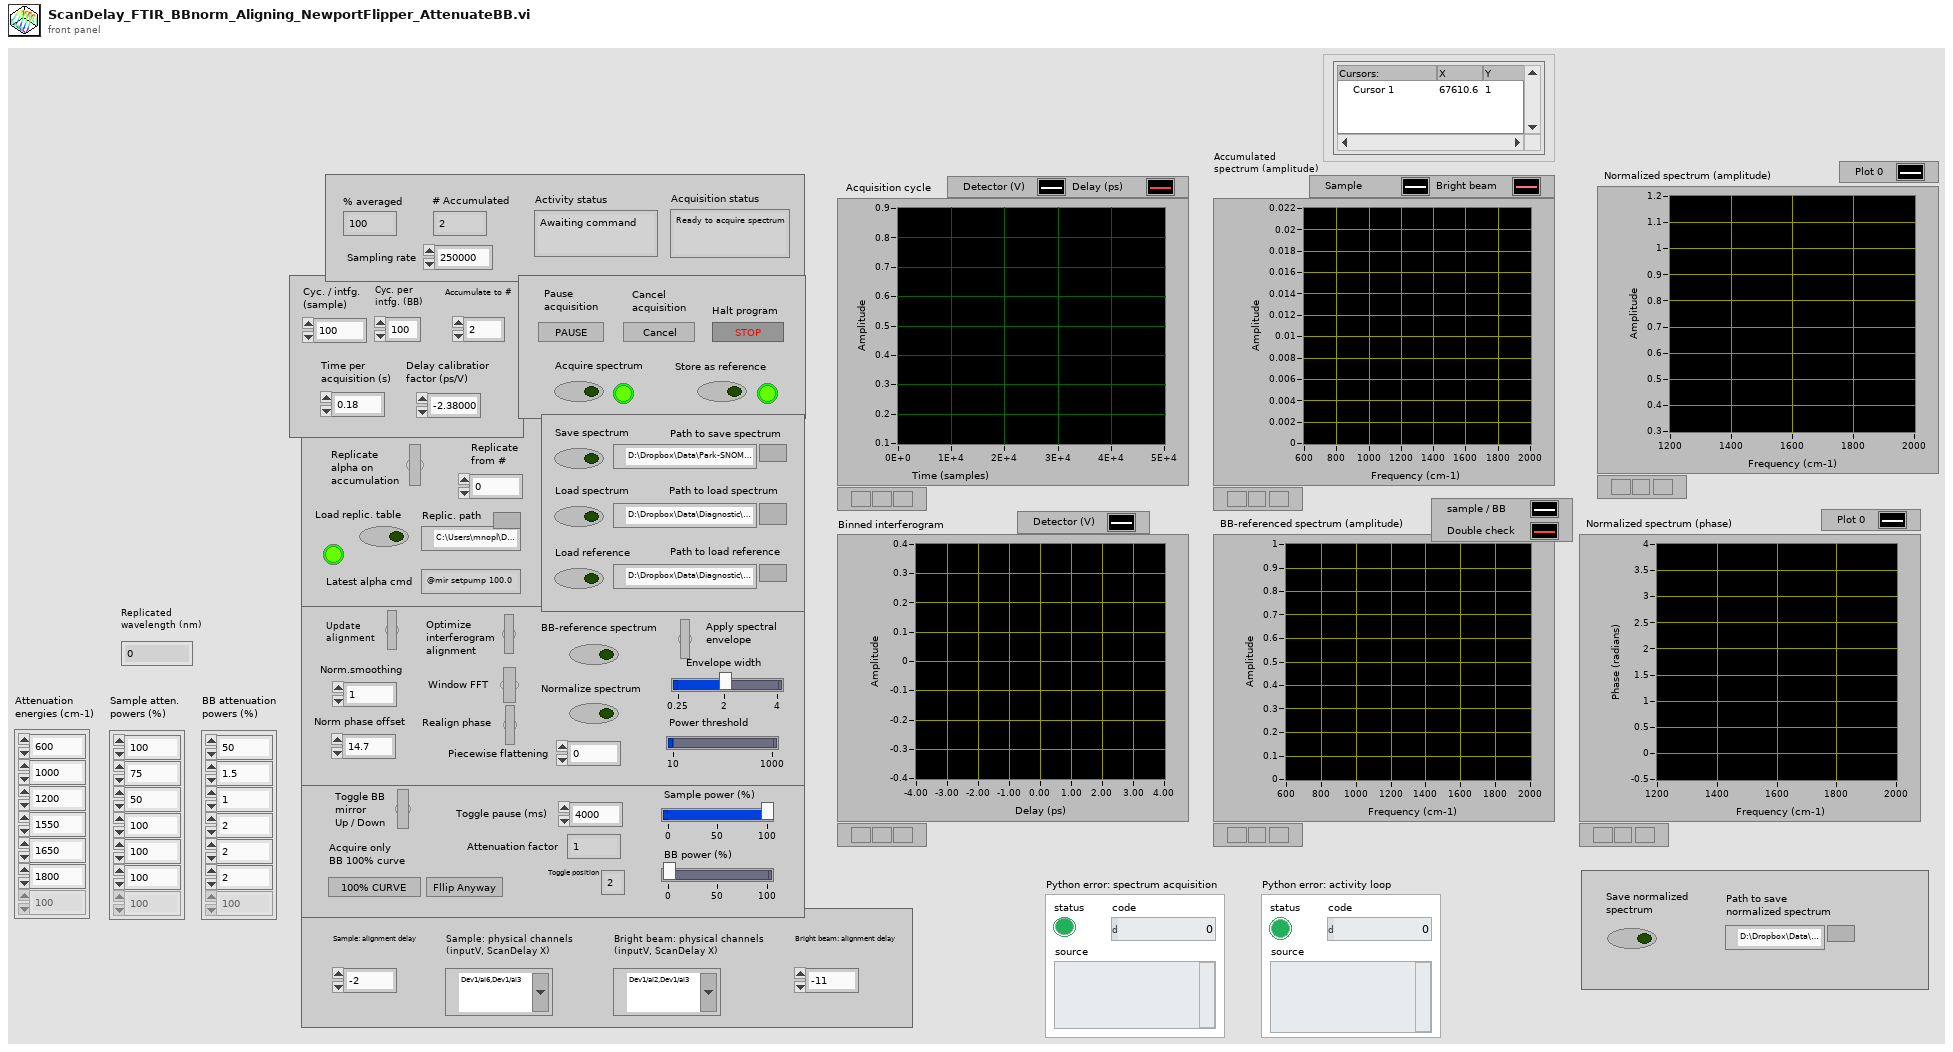
[diagram p1: front panel]
types:
  T1 = cluster{"Output spectrum":dbl[], "Output spectrum":dbl[]}
  T2 = cluster{"Sample Spectra":dbl[], "Sample Spectra":dbl[]}
  T3 = cluster{"Output spectrum":dbl[], "Output spectrum":dbl[]}[]
  T4 = typedef "Control_scanDelayWorkflow.ctl" = enum16{"Initialize", "Sit Idle", "Load replicator table", "Flip BB", "Load Spectrum", "Store reference", "Save Spectrum", "Load reference", "Check Reference", "Check Spectrum", "BB reference spectrum", "Normalize Spectrum", "Save normalized spectrum", "Done"}
  T5 = typedef "imagedata.ctl" = cluster{"image type":i32, "image depth":i32, "image":u8[], "mask":u8[], "colors":u32[], "Rectangle":cluster{"left":i16, "top":i16, "right":i16, "bottom":i16}}
  T6 = typedef "Control_GetSpectrum_BBnorm_AttenuateBB.ctl" = enum16{"Initialize", "Replicate alpha", "Flip in BB", "Attenuate alpha", "Get Spectrum", "Accumulate BB spectrum", "Flip out BB", "Accumulate sample spectrum", "Assess accumulation", "Finalize", "Done"}
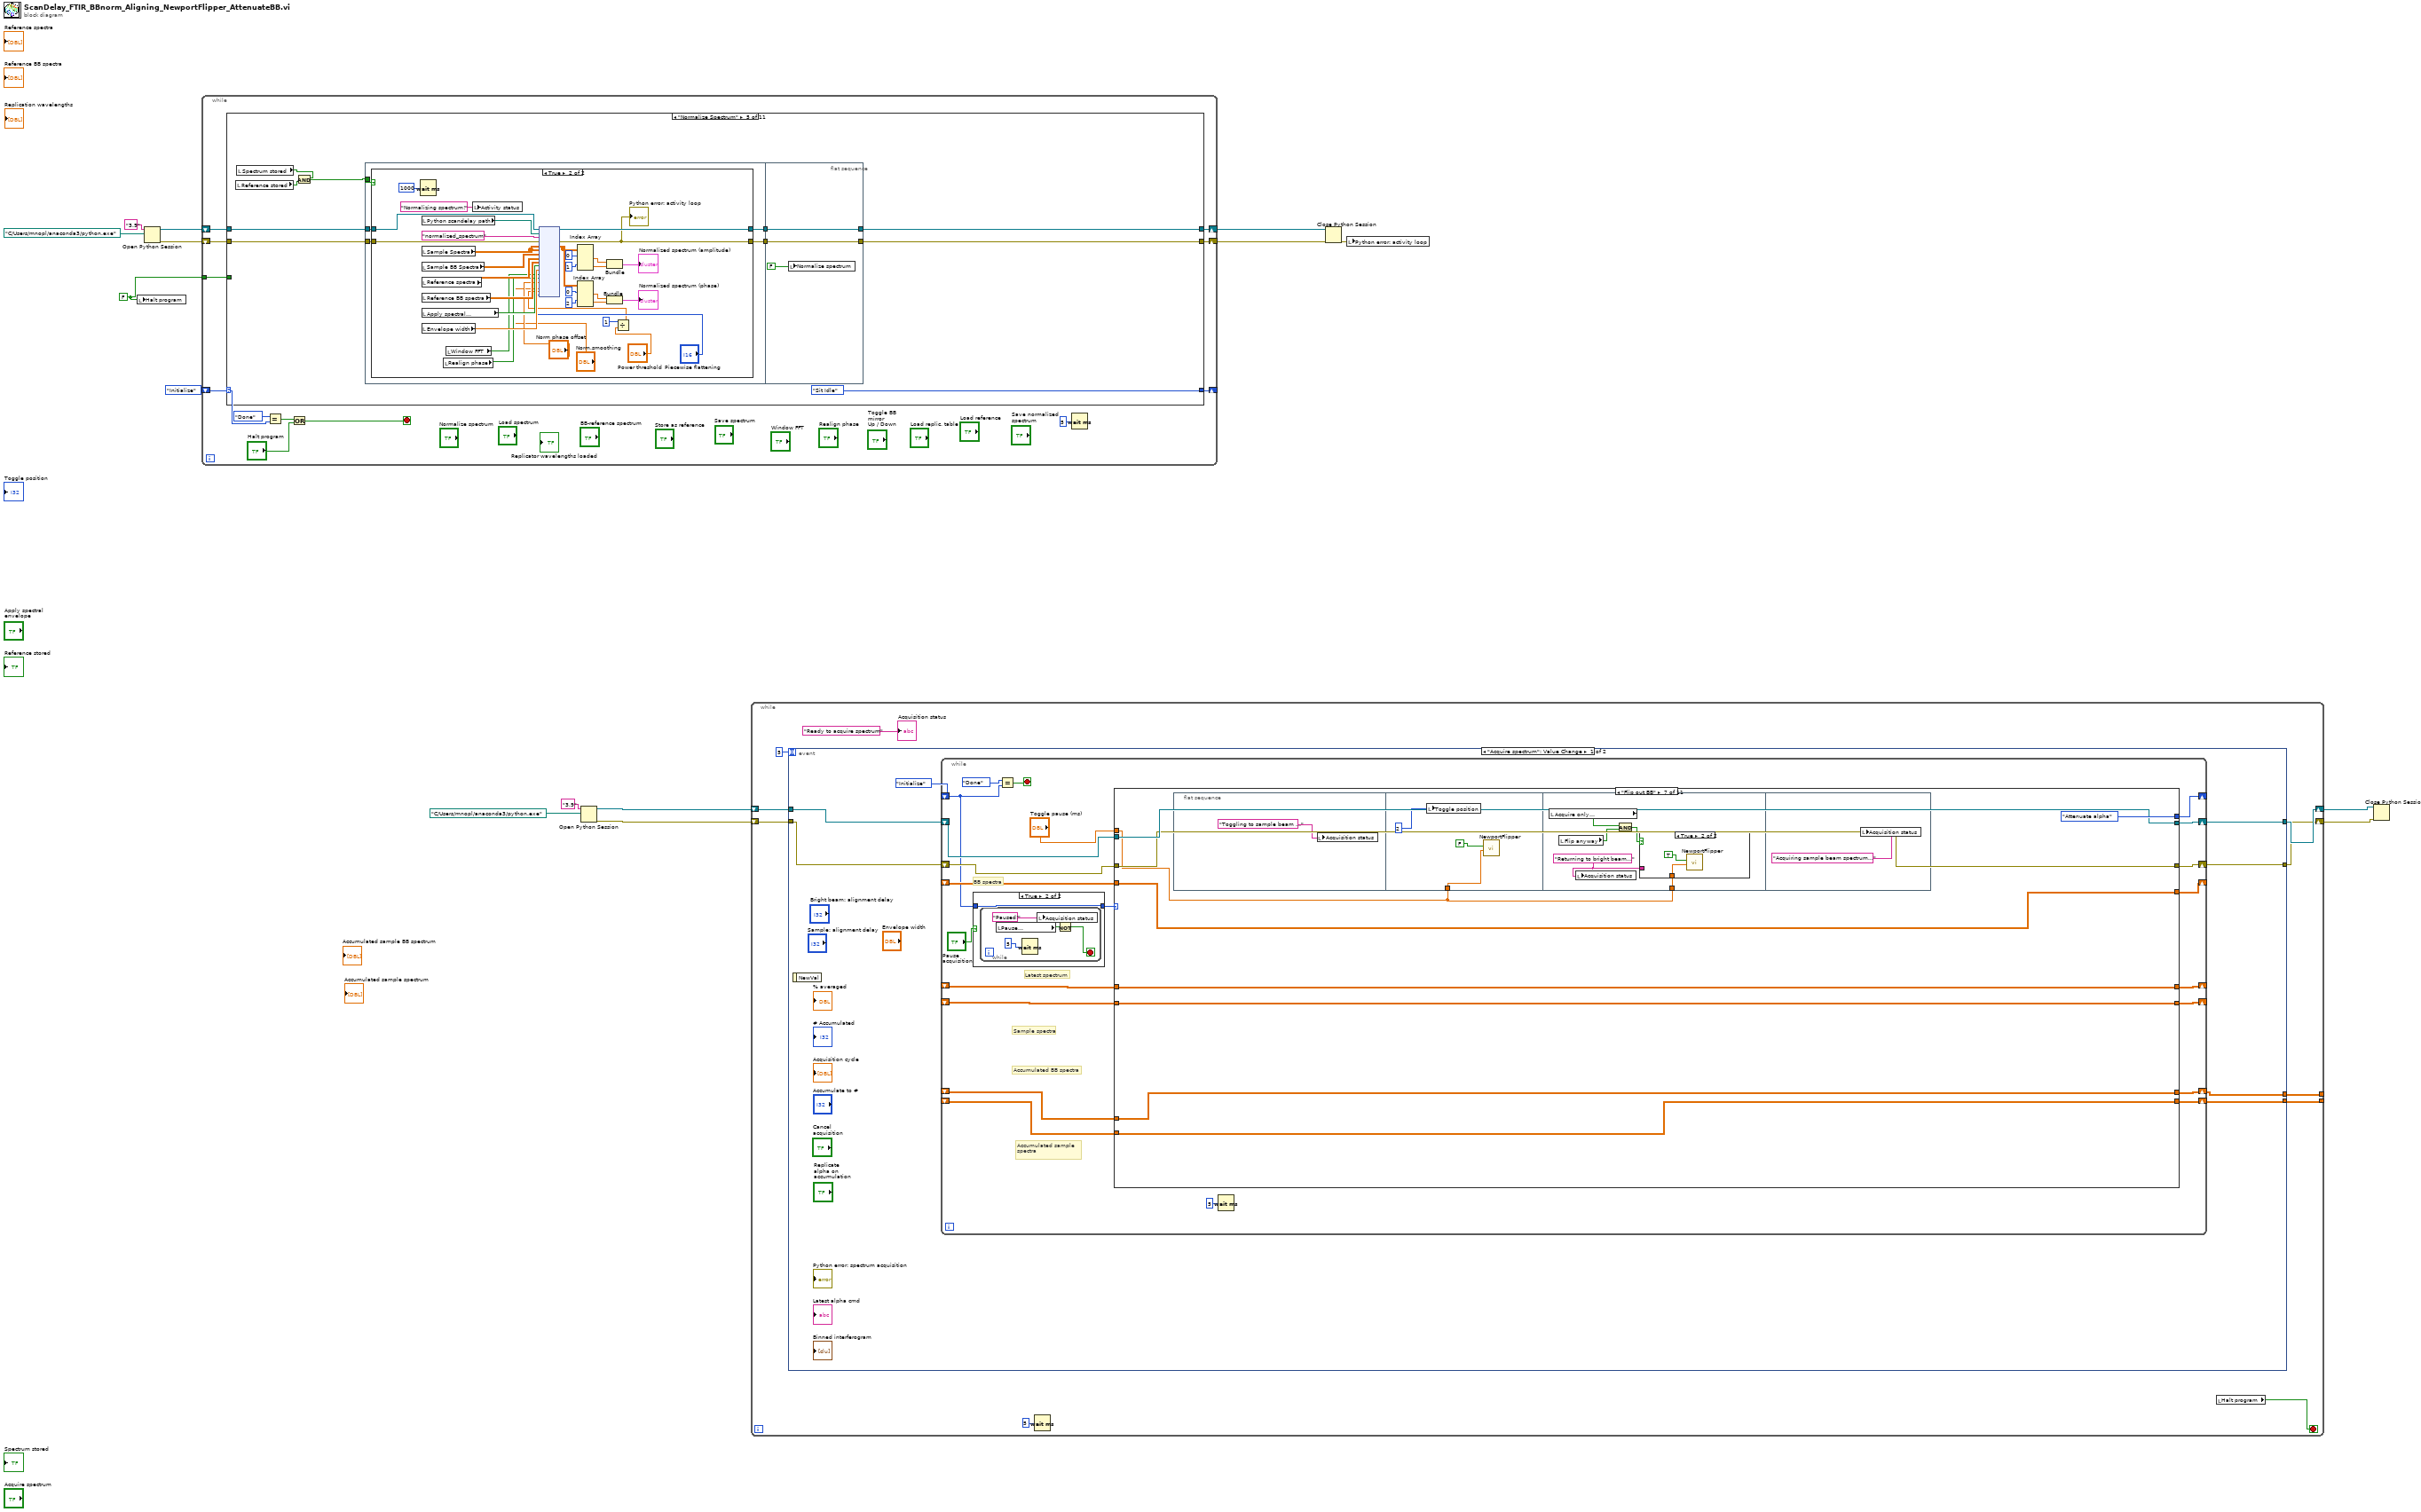
[diagram p0: block diagram]
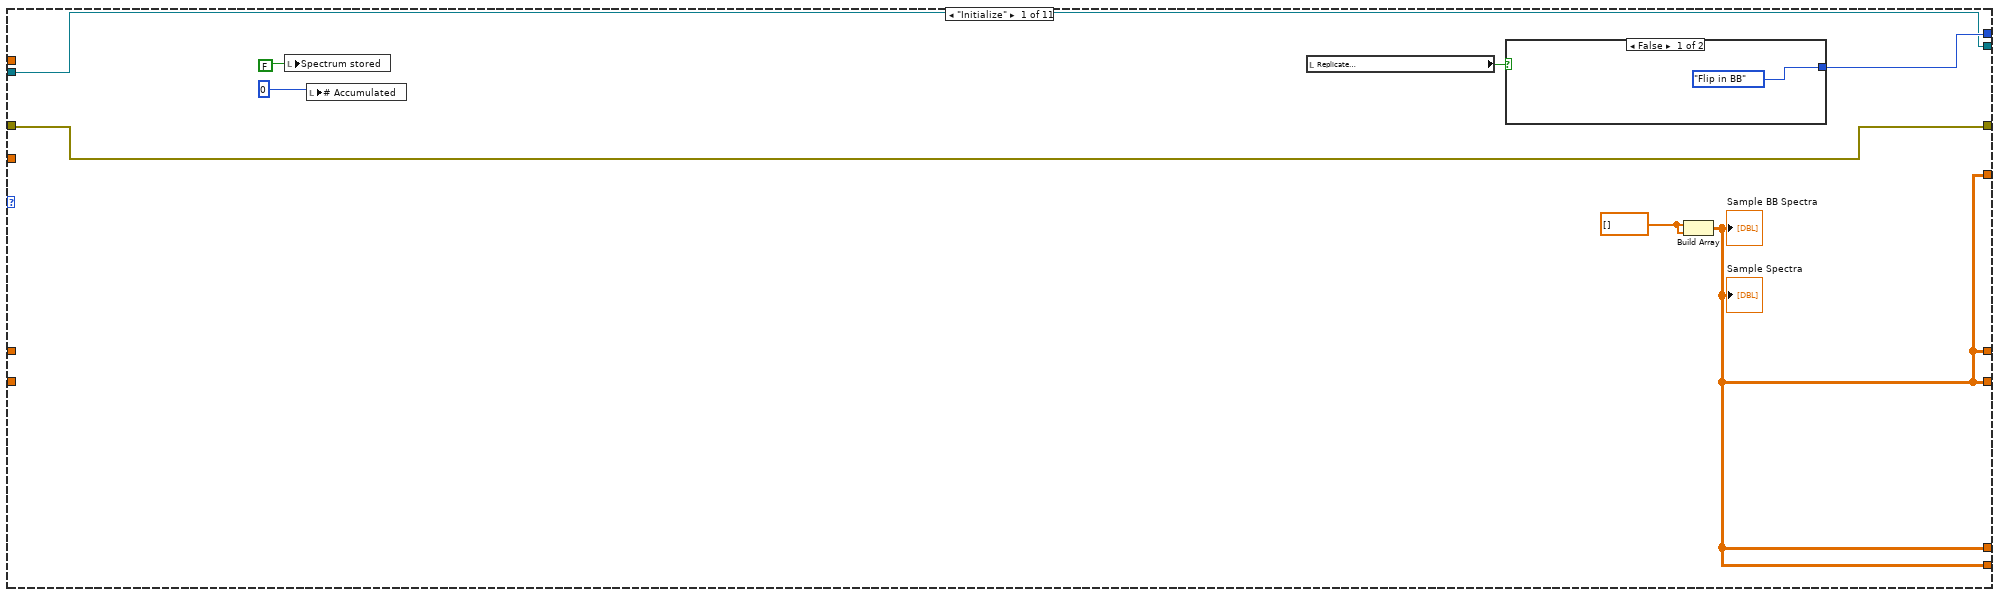
[diagram p3: hidden frame]
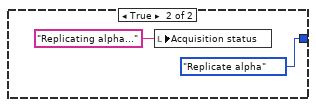
[diagram p4: hidden frame]
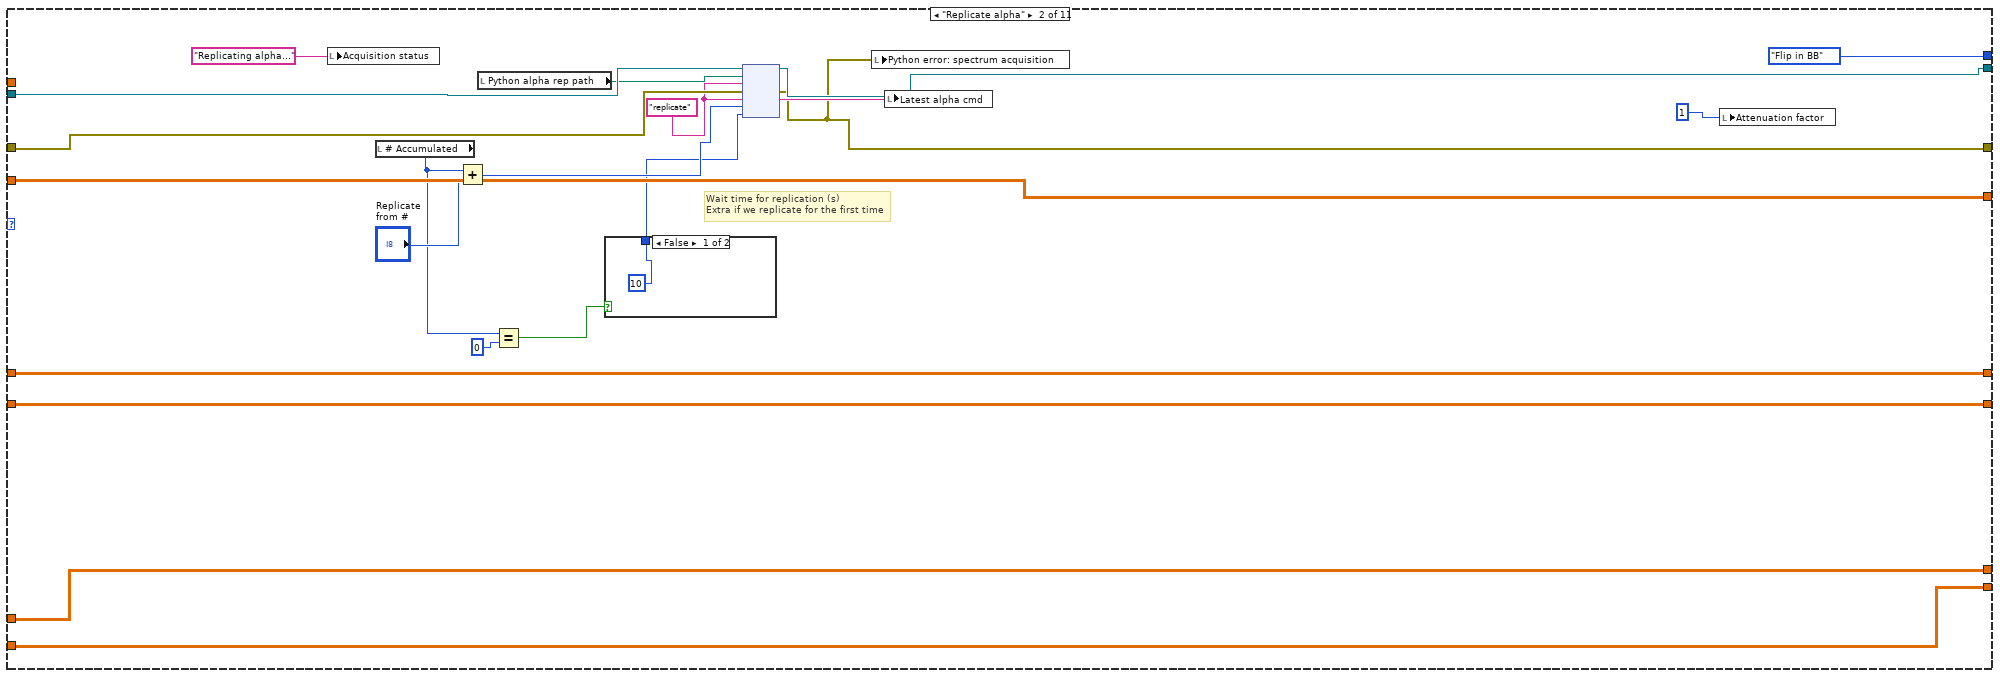
[diagram p5: hidden frame]
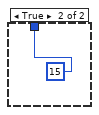
[diagram p6: hidden frame]
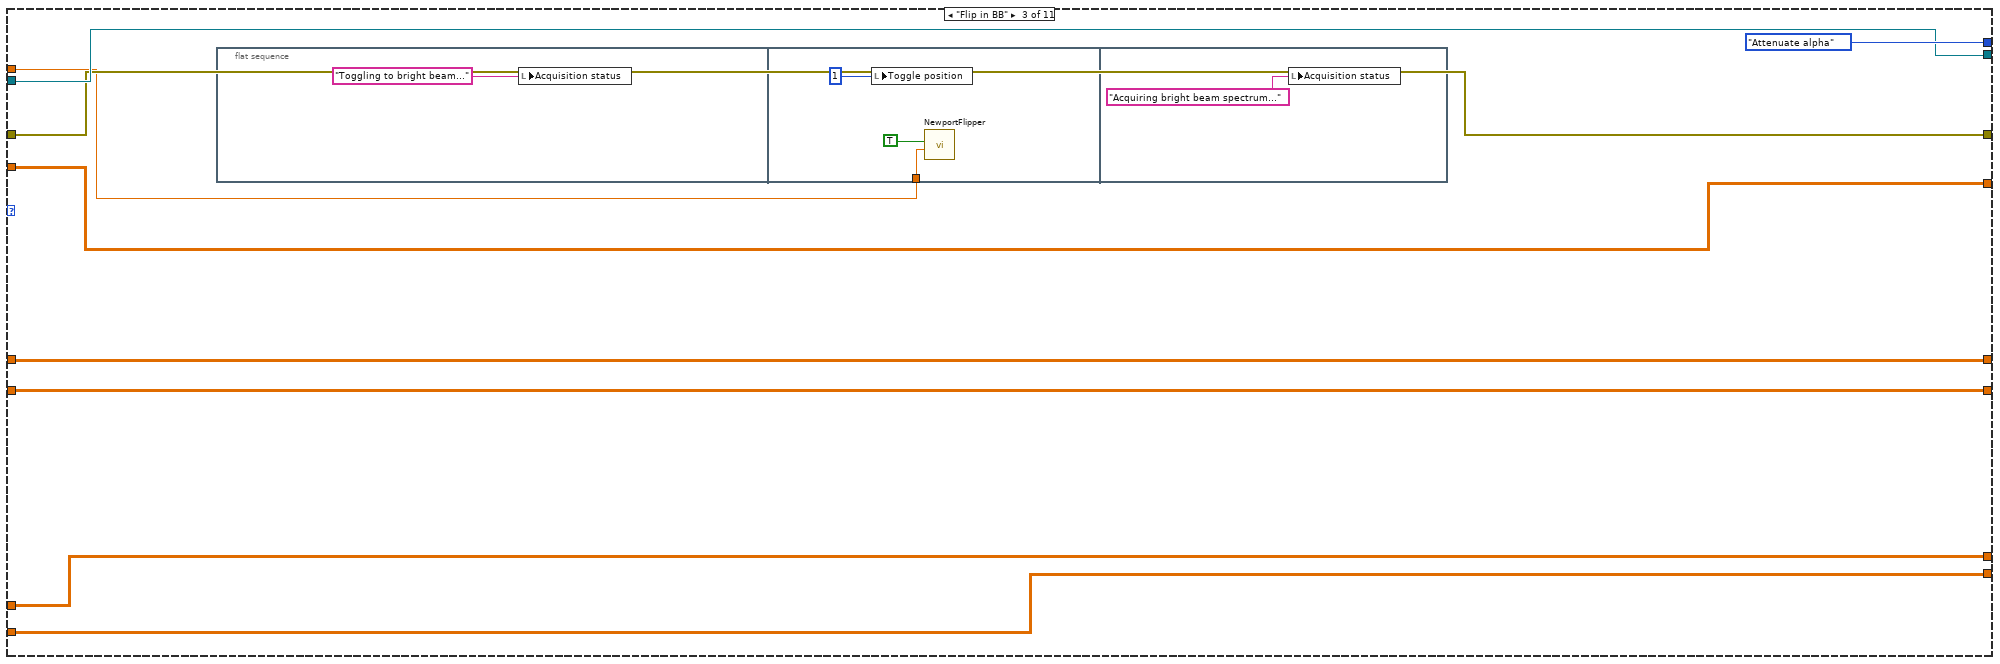
[diagram p7: hidden frame]
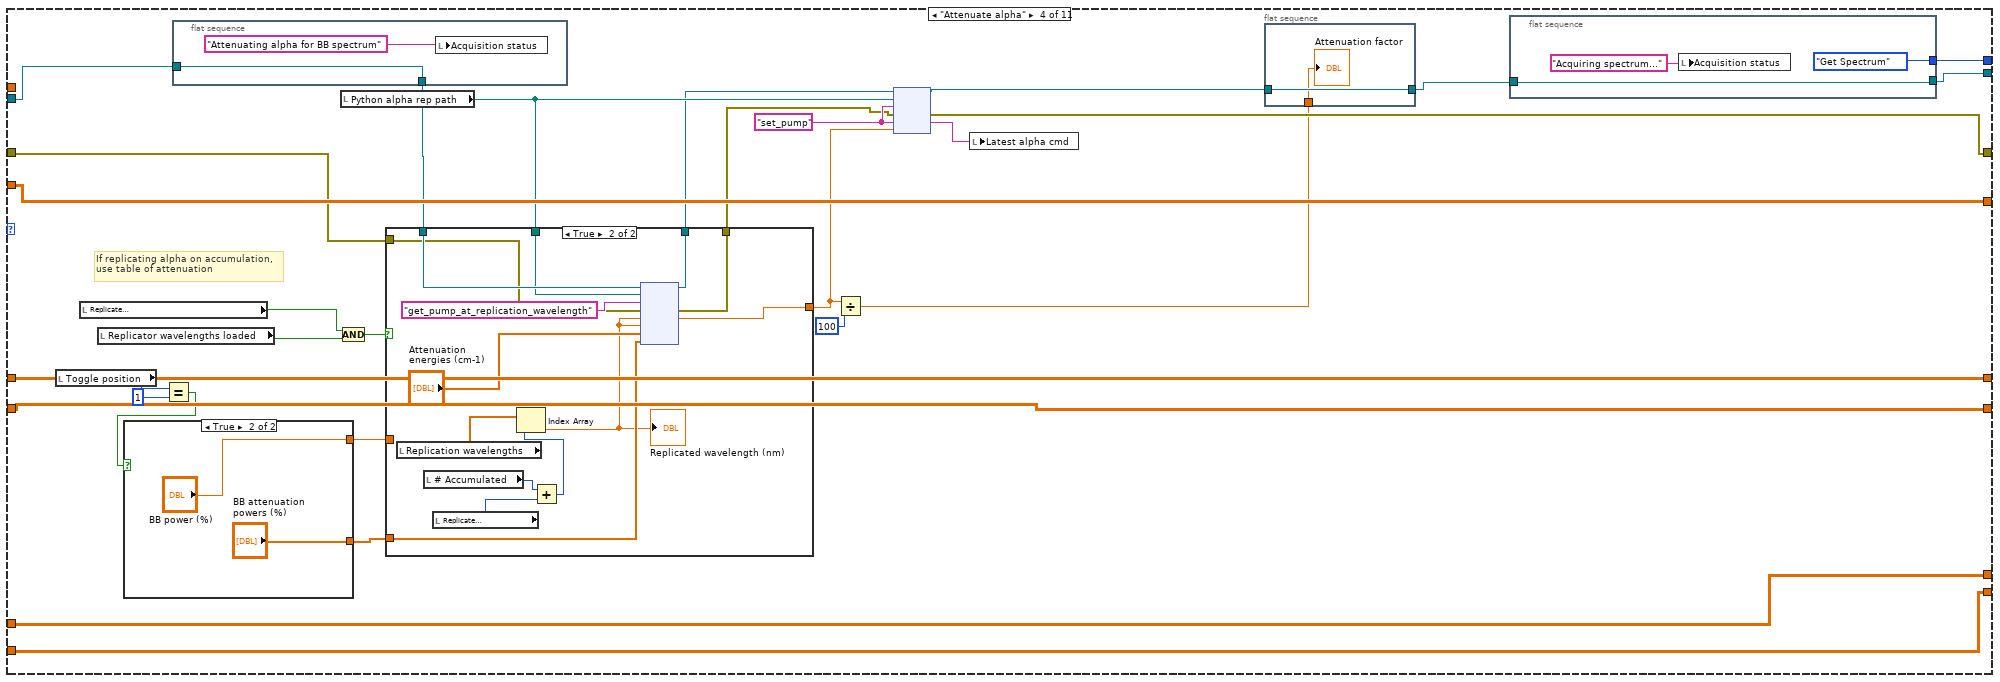
[diagram p8: hidden frame]
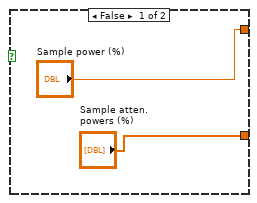
[diagram p9: hidden frame]
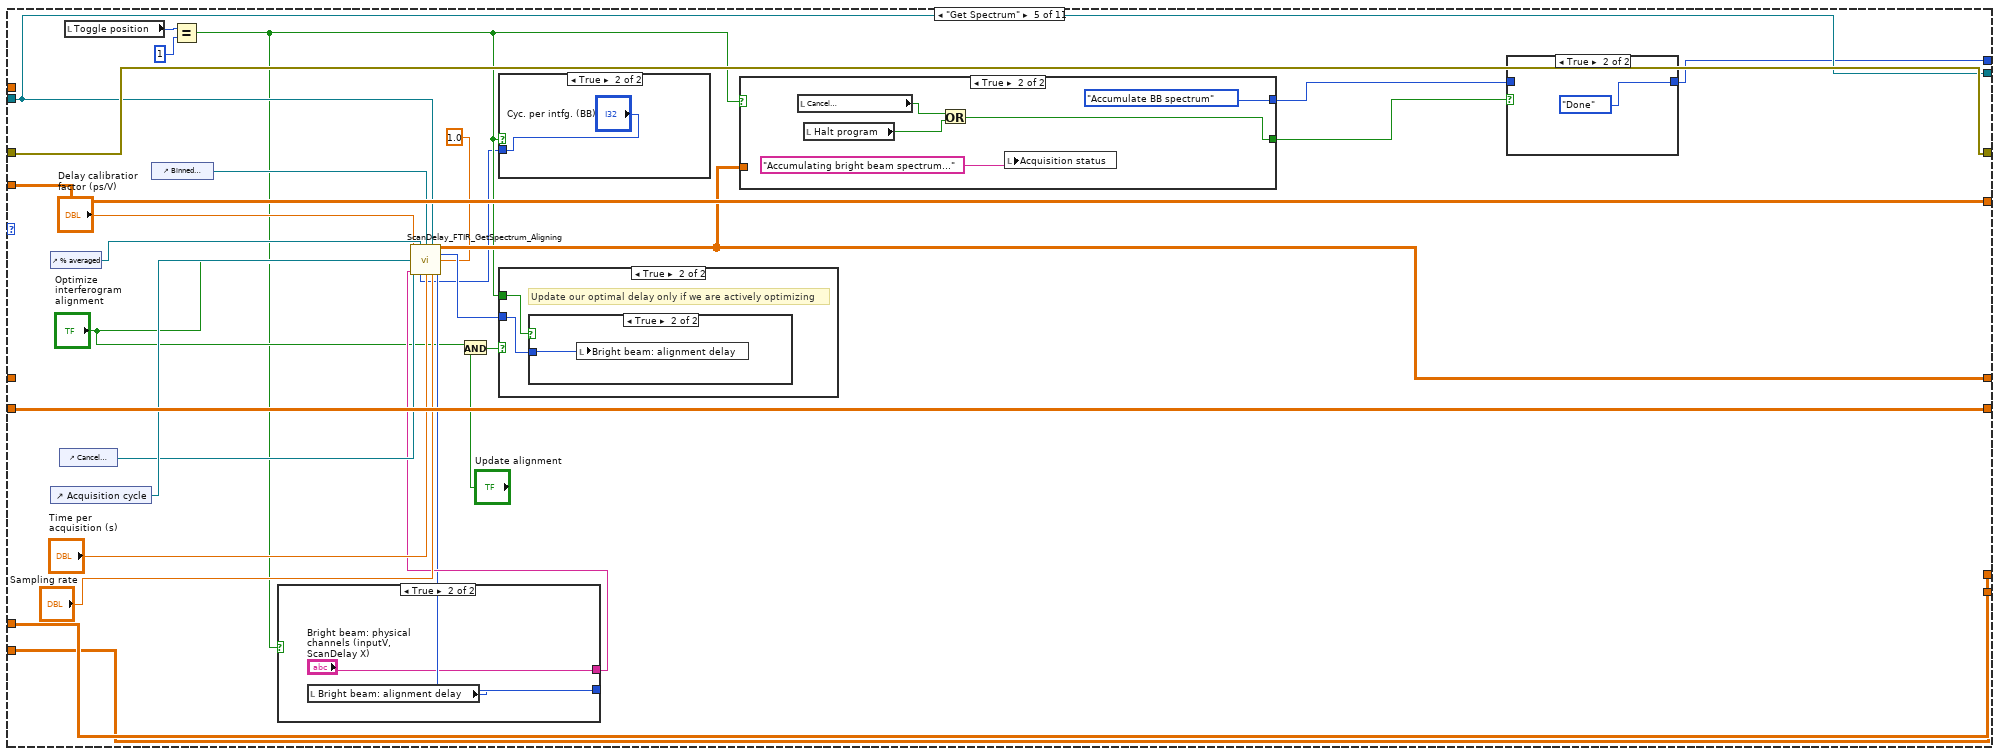
[diagram p11: hidden frame]
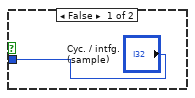
[diagram p12: hidden frame]
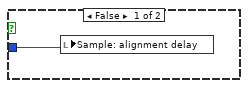
[diagram p14: hidden frame]
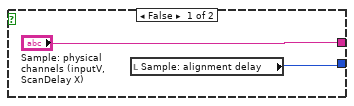
[diagram p15: hidden frame]
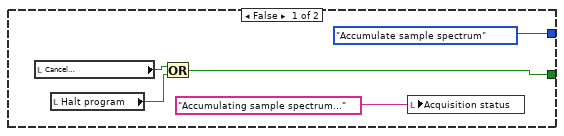
[diagram p17: hidden frame]
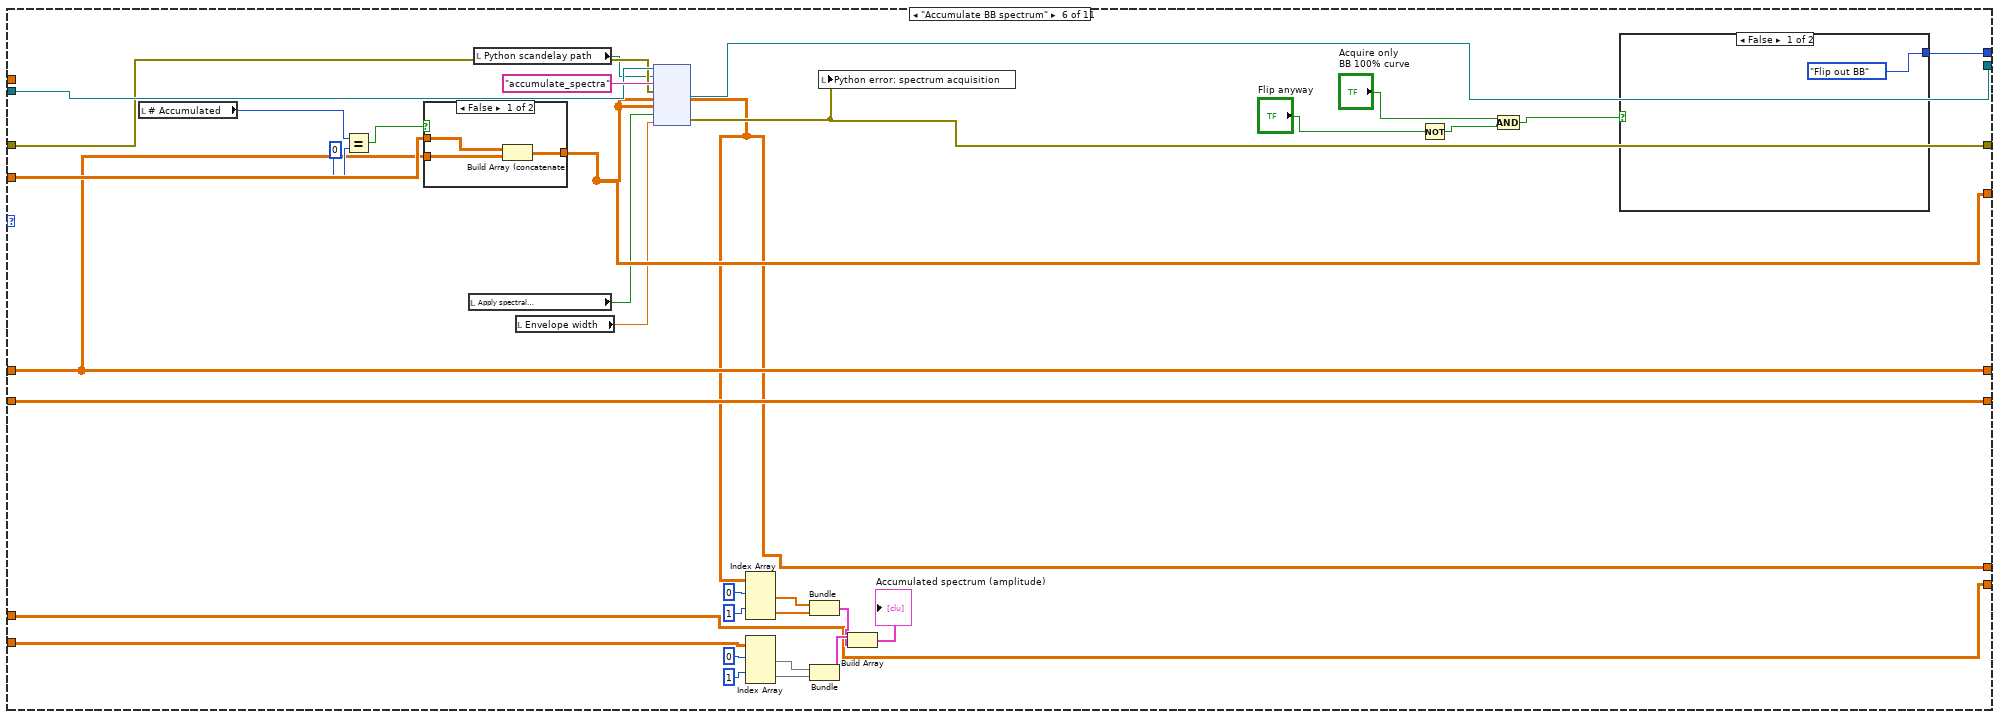
[diagram p18: hidden frame]
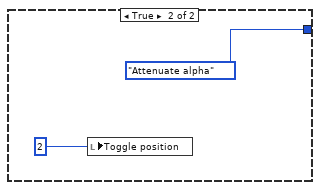
[diagram p19: hidden frame]
diagram:
  w1 = FALSE
  n1 = local write "Halt program"(w1) -> ()
  n2 = Open Python Session(python version="3.9", python path=path "C:/Users/mnopl/anaconda3/python.exe") -> (session out=w11:refnum<k35>, error out=w10:errorcluster)  [unwired: 1 in]
  n3 = while {
    shift-right: [w20] -> _
    shift-left: Control_scanDelayWorkflow."Initialize" -> [w17]
    shift-right: [w26] -> w12
    shift-left: w10 -> [w18]
    shift-right: [w21] -> w13
    shift-left: w11 -> [w19]
    tunnel: w1 -> [w16]
    stop <- w24 stop-if-true
    n4 = case shown="\"Normalize Spectrum\"" w17 {
      tunnel: [w31 w74 w84 w103 w124 w175 w196 w208 w251 w258 w302] -> w26
      tunnel: w19 -> [w32 w73 w83 w104 w127 w176 w197 w206 w252 w259 w303]
      tunnel: w18 -> [w31 w74 w84 w103 w126 w175 w196 w205 w251 w258 w302]
      tunnel: [w32 w73 w83 w104 w125 w176 w197 w207 w252 w259 w303] -> w21
      tunnel: [w30 Control_scanDelayWorkflow."Sit Idle" Control_scanDelayWorkflow."Sit Idle" Control_scanDelayWorkflow."Sit Idle" Control_scanDelayWorkflow."Sit Idle" Control_scanDelayWorkflow."Sit Idle" Control_scanDelayWorkflow."Sit Idle" Control_scanDelayWorkflow."Sit Idle" Control_scanDelayWorkflow."Sit Idle" Control_scanDelayWorkflow."Sit Idle" Control_scanDelayWorkflow."Sit Idle"] -> w20
      tunnel: w16 -> [_ _ _ _ _ _ w193 _ _ _ _]
      frame "Sit Idle", Default {
        n5 = event shown="[5] \"Load replic. table\": Value Change" {
          selector: _ -> [_ _ _ _ _ _ _ _ _ _]
          dyn-events: _ -> [_ _ _ _ _ _ _ _ _ _]
          timeout: 5 -> [_ _ _ _ _ _ _ _ _ w66]
          tunnel: [w33 w37 w44 Control_scanDelayWorkflow."Flip BB" w46 w50 w54 w58 w62 Control_scanDelayWorkflow."Sit Idle"] -> w30
          event "Normalize spectrum": Value Change {
            n6 = event-data() -> ("NewVal"=w34:bool)  [unwired: 1 in]
            n7 = Select(t=Control_scanDelayWorkflow."Normalize Spectrum", s=w34, f=Control_scanDelayWorkflow."Sit Idle") -> (s? t:f=w33:T4)
          }
          event "Store as reference": Value Change {
            n8 = event-data() -> ("NewVal"=w40:bool)  [unwired: 1 in]
            n9 = Select(t=Control_scanDelayWorkflow."Store reference", s=w40, f=Control_scanDelayWorkflow."Sit Idle") -> (s? t:f=w37:T4)
          }
          event "BB-reference spectrum": Value Change {
            n10 = event-data() -> ("NewVal"=w42:bool)  [unwired: 1 in]
            n11 = Select(t=Control_scanDelayWorkflow."BB reference spectrum", s=w42, f=Control_scanDelayWorkflow."Sit Idle") -> (s? t:f=w44:T4)
          }
          event "Toggle BB\nmirror\nUp / Down": Value Change {
            n12 = event-data() -> ()  [unwired: 1 in, 1 out]
          }
          event "Save normalized\nspectrum": Value Change {
            n13 = event-data() -> ("NewVal"=w47:bool)  [unwired: 1 in]
            n14 = Select(t=Control_scanDelayWorkflow."Save normalized spectrum", s=w47, f=Control_scanDelayWorkflow."Sit Idle") -> (s? t:f=w46:T4)
          }
          event "Load replic. table": Value Change {
            n15 = event-data() -> ("NewVal"=w53:bool)  [unwired: 1 in]
            n16 = Select(t=Control_scanDelayWorkflow."Load replicator table", s=w53, f=Control_scanDelayWorkflow."Sit Idle") -> (s? t:f=w50:T4)
          }
          event "Save spectrum": Value Change {
            n17 = event-data() -> ("NewVal"=w55:bool)  [unwired: 1 in]
            n18 = Select(t=Control_scanDelayWorkflow."Save Spectrum", s=w55, f=Control_scanDelayWorkflow."Sit Idle") -> (s? t:f=w54:T4)
          }
          event "Load reference": Value Change {
            n19 = event-data() -> ("NewVal"=w61:bool)  [unwired: 1 in]
            n20 = Select(t=Control_scanDelayWorkflow."Load reference", s=w61, f=Control_scanDelayWorkflow."Sit Idle") -> (s? t:f=w58:T4)
          }
          event "Load spectrum": Value Change {
            n21 = event-data() -> ("NewVal"=w63:bool)  [unwired: 1 in]
            n22 = Select(t=Control_scanDelayWorkflow."Load Spectrum", s=w63, f=Control_scanDelayWorkflow."Sit Idle") -> (s? t:f=w62:T4)
          }
          event Timeout {
            n23 = event-data() -> ()  [unwired: 1 in, 2 out]
            n24 = Wait (ms)(milliseconds to wait=w66) -> ()  [unwired: 1 out]
          }
        }
        "Activity status" <- "Awaiting command"
      }
      frame "Store reference" {
        # "Is spectrum a full array?"
        n25 = local read "Sample Spectra"() -> (w69:dbl[][])
        n26 = local read "Sample BB Spectra"() -> (w68:dbl[][])
        n27 = Empty Array?(array=w69) -> (empty?=w71:bool)
        n28 = Not(x=w71) -> (.not. x?=w70:bool)
        n29 = case shown="True" w70 {
          tunnel: w69 -> [_ w77]
          tunnel: w68 -> [_ w78]
          frame False {
            n30 = Wait (ms)(milliseconds to wait=1000) -> ()  [unwired: 1 out]
            n31 = local write "Activity status"("Error: Spectrum is empty!") -> ()
          }
          frame True {
            n32 = local write "Reference BB spectra"(w78) -> ()
            n33 = local write "Reference spectra"(w77) -> ()
            n34 = local write "Reference stored"(TRUE) -> ()
            n35 = Wait (ms)(milliseconds to wait=1000) -> ()  [unwired: 1 out]
            n36 = local write "Activity status"("Storing reference!") -> ()
          }
        }
      }
      frame "Save Spectrum" {
        n37 = flat-sequence {
          frame #0 {
            w90 = "%g"
            n38 = local read "Sample Spectra"() -> (w92:dbl[][])
            n39 = Path To String(path="Path to save spectrum") -> (string=w94:string)
            n40 = local read "Sample BB Spectra"() -> (w85:dbl[][])
            n41 = Search and Replace String(input string=w94, search string="(.txt)*$", replace string=".txt") -> (result string=w98:string)  [unwired: 5 in, 3 out]
            n42 = Search and Replace String(input string=w98, search string=".txt$", replace string="_BB.txt") -> (result string=w97:string)  [unwired: 5 in, 3 out]
            n43 = String To Path(string=w98) -> (path=w95:path)
            n44 = Array To Spreadsheet String(array=w92, 3:w90) -> (spreadsheet string=w91:string)  [unwired: 1 in]
            n45 = Array To Spreadsheet String(array=w85, 3:w90) -> (spreadsheet string=w99:string)  [unwired: 1 in]
            n46 = String To Path(string=w97) -> (path=w96:path)
            n47 = Write to Text File(file (use dialog)=w95, text=w91) -> ()  [unwired: 2 in, 3 out]
            n48 = Write to Text File(file (use dialog)=w96, text=w99) -> ()  [unwired: 2 in, 3 out]
          }
          frame #1 {
            n49 = local write "Activity status"("Successfully saved spectrum!") -> ()
            n50 = Wait (ms)(milliseconds to wait=1000) -> ()  [unwired: 1 out]
          }
        }
      }
      frame "Load reference" {
        n51 = flat-sequence {
          frame #0 {
            w109 = "%g"
            n52 = Path To String(path="Path to load reference") -> (string=w105:string)
            n53 = Search and Replace String(input string=w105, search string=".txt$", replace string="_BB.txt") -> (result string=w107:string)  [unwired: 5 in, 3 out]
            n54 = Read from Text File(file (use dialog)="Path to load reference") -> (text=w110:string)  [unwired: 3 in, 3 out]
            n55 = String To Path(string=w107) -> (path=w114:path)
            n56 = Spreadsheet String To Array(format string=w109, spreadsheet string=w110) -> (array=w111:dbl[][])  [unwired: 2 in]
            n57 = Read from Text File(file (use dialog)=w114) -> (text=w113:string)  [unwired: 3 in, 3 out]
            n58 = local write "Reference spectra"(w111) -> ()
            n59 = Spreadsheet String To Array(format string=w109, spreadsheet string=w113) -> (array=w115:dbl[][])  [unwired: 2 in]
            n60 = local write "Reference BB spectra"(w115) -> ()
          }
          frame #1 {
            n61 = local write "Reference stored"(TRUE) -> ()
            n62 = Wait (ms)(milliseconds to wait=1000) -> ()  [unwired: 1 out]
            n63 = local write "Activity status"("Successfully loaded reference!") -> ()
          }
        }
      }
      frame "Normalize Spectrum" {
        n64 = local read "Reference stored"() -> (w121:bool)
        n65 = local read "Spectrum stored"() -> (w120:bool)
        n66 = And(x=w120, y=w121) -> (x .and. y?=w119:bool)
        n67 = flat-sequence {
          tunnel: w127 -> [w133]
          tunnel: w126 -> [w132]
          tunnel: [w131] -> w123
          tunnel: [w130] -> w122
          tunnel: w119 -> [w129]
          tunnel: [w172] -> w124
          tunnel: [w173] -> w125
          tunnel: w123 -> [w173]
          tunnel: w122 -> [w172]
          frame #0 {
            n68 = case shown="True" w129 {
              tunnel: w133 -> [w135 w169]
              tunnel: w132 -> [w134 w168]
              tunnel: [w135 w167] -> w131
              tunnel: [w134 w150] -> w130
              frame False {
                n69 = Wait (ms)(milliseconds to wait=1000) -> ()  [unwired: 1 out]
                n70 = local write "Activity status"("Error: Spectrum or reference is empty!") -> ()
              }
              frame True {
                n71 = Wait (ms)(milliseconds to wait=1000) -> ()  [unwired: 1 out]
                n72 = local read "Python scandelay path"() -> (w166:path)
                n73 = local read "Sample Spectra"() -> (w151:dbl[][])
                n74 = local read "Sample BB Spectra"() -> (w152:dbl[][])
                n75 = local read "Reference spectra"() -> (w149:dbl[][])
                n76 = local read "Reference BB spectra"() -> (w148:dbl[][])
                n77 = local read "Apply spectral\nenvelope"() -> (w147:bool)
                n78 = local read "Envelope width"() -> (w146:dbl)
                n79 = local read "Realign phase"() -> (w144:bool)
                n80 = local read "Window FFT"() -> (w145:bool)
                n81 = local write "Activity status"("Normalizing spectrum!") -> ()
                n82 = Divide(x=1, y="Power threshold") -> (x/y=w139:dbl)
                n83 = node(w169, w166, "normalized_spectrum", w168, w151, w151, w152, w149, w148, w147, w146, w145, w144, "Norm phase offset", "Norm.smoothing", w139, "Piecewise flattening") -> (w167:refnum<k35>, w150:errorcluster, w154:dbl[][])  [unwired: 12 in, 2 out]
                "Python error: activity loop" <- w150
                n84 = Index Array(array=w154, index (row) #1=0, index (row) #2=1) -> (element #1=w162:dbl[], element #2=w161:dbl[])  [unwired: 2 in]
                n85 = Index Array(array=w154, index (row) #1=0, index (row) #2=2) -> (element #1=w158:dbl[], element #2=w157:dbl[])  [unwired: 2 in]
                n86 = Bundle("Sample Spectra"=w162, "Sample Spectra"=w161) -> (→"Normalized spectrum (amplitude)":T2)  [unwired: 1 in]
                n87 = Bundle("Sample Spectra"=w158, "Sample Spectra"=w157) -> (→"Normalized spectrum (phase)":T2)  [unwired: 1 in]
              }
            }
          }
          frame #1 {
            n88 = local write "Normalize spectrum"(FALSE) -> ()
          }
        }
      }
      frame "Load Spectrum" {
        n89 = flat-sequence {
          frame #0 {
            w184 = "%g"
            n90 = Path To String(path="Path to load spectrum") -> (string=w180:string)
            n91 = Search and Replace String(input string=w180, search string=".txt$", replace string="_BB.txt") -> (result string=w182:string)  [unwired: 5 in, 3 out]
            n92 = Read from Text File(file (use dialog)="Path to load spectrum") -> (text=w185:string)  [unwired: 3 in, 3 out]
            n93 = String To Path(string=w182) -> (path=w187:path)
            n94 = Spreadsheet String To Array(format string=w184, spreadsheet string=w185) -> (array=w178:dbl[][])  [unwired: 2 in]
            n95 = Read from Text File(file (use dialog)=w187) -> (text=w186:string)  [unwired: 3 in, 3 out]
            n96 = Spreadsheet String To Array(format string=w184, spreadsheet string=w186) -> (array=w177:dbl[][])  [unwired: 2 in]
            n97 = local write "Sample Spectra"(w178) -> ()
            n98 = local write "Sample BB Spectra"(w177) -> ()
          }
          frame #1 {
            n99 = local write "Load spectrum"(FALSE) -> ()
            n100 = local write "Spectrum stored"(TRUE) -> ()
            n101 = local write "Activity status"("Successfully loaded spectrum!") -> ()
            n102 = Wait (ms)(milliseconds to wait=1000) -> ()  [unwired: 1 out]
          }
        }
      }
      frame "Initialize" {
        # "Fine so long as we've saved default values for \"replication wavelengths\""
        n103 = local write "Replicator wavelengths loaded"(TRUE) -> ()
        n104 = local write "Reference stored"(w193) -> ()
        n105 = local write "Spectrum stored"(w193) -> ()
        n106 = local write "Acquire spectrum"(w193) -> ()
        "Python scandelay path" <- path "C:/Users/mnopl/Desktop/software/mnOPSuite/PRISM/python/scandelay_FTIR.py"
        "Python alpha rep path" <- path "C:/Users/mnopl/Desktop/software/mnOPSuite/PRISM/python/alpha.py"
      }
      frame "BB reference spectrum" {
        # "Is spectrum a full array?"
        n107 = local read "Sample Spectra"() -> (w199:dbl[][])
        n108 = Empty Array?(array=w199) -> (empty?=w201:bool)
        n109 = Not(x=w201) -> (.not. x?=w200:bool)
        n110 = flat-sequence {
          tunnel: w206 -> [w212]
          tunnel: w205 -> [w211]
          tunnel: w200 -> [w210]
          tunnel: [w214] -> w203
          tunnel: [w213] -> w202
          tunnel: w199 -> [w209]
          tunnel: [w248] -> w207
          tunnel: [w249] -> w208
          tunnel: w203 -> [w249]
          tunnel: w202 -> [w248]
          frame #0 {
            n111 = case shown="True" w210 {
              tunnel: [w215 w226] -> w214
              tunnel: [w216 w227] -> w213
              tunnel: w212 -> [w216 w236]
              tunnel: w211 -> [w215 w235]
              tunnel: w209 -> [_ w231]
              frame False {
                n112 = Wait (ms)(milliseconds to wait=1000) -> ()  [unwired: 1 out]
                n113 = local write "Activity status"("Error: Spectrum or reference is empty!") -> ()
              }
              frame True {
                n114 = local read "Python scandelay path"() -> (w230:path)
                n115 = local read "Sample BB Spectra"() -> (w234:dbl[][])
                n116 = local read "Apply spectral\nenvelope"() -> (w225:bool)
                n117 = local read "Envelope width"() -> (w224:dbl)
                n118 = local read "Realign phase"() -> (w222:bool)
                n119 = local read "Window FFT"() -> (w223:bool)
                n120 = Wait (ms)(milliseconds to wait=1000) -> ()  [unwired: 1 out]
                n121 = local write "Activity status"("Referencing spectrum to bright beam...") -> ()
                n122 = local read "Power threshold"() -> (w220:dbl)
                n123 = Divide(x=1, y=w220) -> (x/y=w219:dbl)
                n124 = node(w236, w230, "BB_referenced_spectrum", w235, w231, w231, w234, w225, w224, w223, w222, w219) -> (w227:refnum<k35>, w226:errorcluster, w241:dbl[][])  [unwired: 7 in, 2 out]
                n125 = local write "Python error: activity loop"(w226) -> ()
                n126 = Index Array(array=w241, index (row) #1=0, index (row) #2=2) -> (element #1=w244:dbl[], element #2=w243:dbl[])  [unwired: 2 in]
                n127 = Index Array(array=w241, index (row) #1=0, index (row) #2=1) -> (element #1=w246:dbl[], element #2=w245:dbl[])  [unwired: 2 in]
                n128 = Bundle("Sample Spectra"=w244, "Sample Spectra"=w243) -> (→"BB-referenced spectrum (phase)":T2)  [unwired: 1 in]
                n129 = Bundle("Sample Spectra"=w246, "Sample Spectra"=w245) -> (→"BB-referenced spectrum (amplitude)":T2)  [unwired: 1 in]
              }
            }
          }
          frame #1 {
            n130 = local write "BB-reference spectrum"(FALSE) -> ()
          }
        }
      }
      frame "Flip BB" {
        n131 = local read "Toggle BB\nmirror\nUp / Down"() -> (w254:bool)
        n132 = local read "Toggle pause (ms)"() -> (w250:dbl)
        n133 = call "NewportFlipper.vi"("Settle time (ms)"=w250, "Up/Down"=w254) -> ()  [unwired: 10 in]
      }
      frame "Save normalized spectrum" {
        n134 = flat-sequence {
          tunnel: [w273] -> w260
          tunnel: [w261] -> w255
          tunnel: w260 -> [w287]
          tunnel: [w284] -> w256
          tunnel: w255 -> [w284]
          tunnel: w256 -> [w296]
          frame #0 {
            w278 = "%g"
            n135 = Path To String(path="Path to save\nnormalized spectrum") -> (string=w273:string)
            n136 = property on="Normalized spectrum (phase)" class="XYGraph (strict)"() -> ("Value"=w263:T1)  [unwired: 2 in, 2 out]
            n137 = property on="Normalized spectrum (amplitude)" class="XYGraph (strict)"() -> ("Value"=w271:T1)  [unwired: 2 in, 2 out]
            n138 = Unbundle(w271) -> ("Output spectrum"=w270:dbl[], "Output spectrum"=w269:dbl[])
            n139 = Unbundle(w263) -> ("Output spectrum"=w266:dbl[], "Output spectrum"=w265:dbl[])
            n140 = Build Array(w270, w269) -> (w268:dbl[][])
            n141 = Build Array(w266, w265) -> (w264:dbl[][])
            n142 = Search and Replace String(input string=w273, search string="(.txt)$", replace string="_normalized_phase.txt") -> (result string=w282:string)  [unwired: 5 in, 3 out]
            n143 = Search and Replace String(input string=w273, search string="(.txt)*$", replace string="_normalized_amplitude.txt") -> (result string=w261:string)  [unwired: 5 in, 3 out]
            n144 = Transpose 2D Array(2D array=w268) -> (transposed array=w267:dbl[][])
            n145 = Transpose 2D Array(2D array=w264) -> (transposed array=w262:dbl[][])
            n146 = Array To Spreadsheet String(array=w267, 3:w278) -> (spreadsheet string=w283:string)  [unwired: 1 in]
            n147 = Array To Spreadsheet String(array=w262, 3:w278) -> (spreadsheet string=w279:string)  [unwired: 1 in]
            n148 = String To Path(string=w282) -> (path=w281:path)
            n149 = String To Path(string=w261) -> (path=w280:path)
            n150 = Write to Text File(file (use dialog)=w281, text=w283) -> ()  [unwired: 2 in, 3 out]
            n151 = Write to Text File(file (use dialog)=w280, text=w279) -> ()  [unwired: 2 in, 3 out]
          }
          frame #1 {
            n152 = invoke on="Normalized spectrum (amplitude)" class="XYGraph (strict)" method="Get Image"() -> ("image data"=w286:T5)  [unwired: 6 in, 5 out]
            n153 = Search and Replace String(input string=w287, search string="(.txt)$", replace string="_normalized_amplitude.png") -> (result string=w293:string)  [unwired: 5 in, 3 out]
            n154 = String To Path(string=w293) -> (path=w292:path)
            n155 = call <vilib>:"Write PNG File.vi"("image data"=w286, "path to PNG file"=w292) -> ()  [unwired: 8 in, 2 out]
            n156 = invoke on="Normalized spectrum (phase)" class="XYGraph (strict)" method="Get Image"() -> ("image data"=w285:T5)  [unwired: 6 in, 5 out]
            n157 = Search and Replace String(input string=w287, search string="(.txt)$", replace string="_normalized_phase.png") -> (result string=w289:string)  [unwired: 5 in, 3 out]
            n158 = String To Path(string=w289) -> (path=w288:path)
            n159 = call <vilib>:"Write PNG File.vi"("image data"=w285, "path to PNG file"=w288) -> ()  [unwired: 8 in, 2 out]
          }
          frame #2 {
            n160 = local write "Save normalized\nspectrum"(FALSE) -> ()
            n161 = Concatenate Strings("Spectrum successfully saved to:" ("message"), "\r", w296) -> (w299:string)
            n162 = One Button Dialog(message=w299, button name ("OK")="OK") -> ()  [unwired: 1 out]
          }
        }
      }
      frame "Load replicator table" {
        n163 = flat-sequence {
          frame #0 {
            # "A leading whitespace in replication table requires skipping an extra column"
            n164 = Read from Text File(file (use dialog)="Replic. path") -> (text=w311:string)  [unwired: 3 in, 3 out]
            n165 = Spreadsheet String To Array(delimiter (Tab)=" ", format string="%g", spreadsheet string=w311) -> (array=w308:dbl[][])  [unwired: 1 in]
            n166 = Index Array(array=w308, index (col)=4) -> (element=w306:dbl[])  [unwired: 1 in]
            n167 = local write "Replication wavelengths"(w306) -> ()
          }
          frame #1 {
            n168 = local write "Load replic. table"(FALSE) -> ()
            n169 = local write "Replicator wavelengths loaded"(TRUE) -> ()
            n170 = Wait (ms)(milliseconds to wait=1000) -> ()  [unwired: 1 out]
            n171 = local write "Activity status"("Successfully loaded replication wavelengths!") -> ()
          }
        }
      }
    }
    n172 = Equal?(x=Control_scanDelayWorkflow."Done", y=w17) -> (x = y?=w22:bool)
    n173 = Or(x=w22, y="Halt program") -> (x .or. y?=w24:bool)
    n174 = Wait (ms)(milliseconds to wait=5) -> ()  [unwired: 1 out]
  }
  n175 = Open Python Session(python version="3.9", python path=path "C:/Users/mnopl/anaconda3/python.exe") -> (session out=w5:refnum<k35>, error out=w4:errorcluster)  [unwired: 1 in]
  n176 = while {
    shift-right: [w318] -> w2
    shift-left: w4 -> [w320]
    shift-right: [w319] -> w3
    shift-left: w5 -> [w321]
    tunnel: [w317] -> _
    tunnel: [w316] -> _
    stop <- w325 stop-if-true
    n177 = event shown="[0] \"Acquire spectrum\": Value Change" {
      selector: _ -> [_ _]
      dyn-events: _ -> [_ _]
      timeout: 5 -> [_ w657]
      tunnel: w321 -> [w331 w656]
      tunnel: w320 -> [w330 w655]
      tunnel: [w329 w656] -> w319
      tunnel: [w328 w655] -> w318
      tunnel: [w327 _] -> w317
      tunnel: [w326 _] -> w316
      event "Acquire spectrum": Value Change {
        n178 = event-data() -> ()  [unwired: 1 in, 1 out]
        n179 = while {
          shift-right: [w352] -> _
          shift-left: _ -> [w351]
          shift-right: [w353] -> _
          shift-left: _ -> [w350]
          shift-right: [w349] -> _
          shift-left: Control_GetSpectrum_BBnorm_AttenuateBB."Initialize" -> [w335]
          shift-right: [w346] -> w328
          shift-left: w330 -> [w347]
          shift-right: [w345] -> w329
          shift-left: w331 -> [w348]
          shift-right: [w344] -> _
          shift-left: _ -> [w342]
          shift-right: [w340] -> w327
          shift-left: _ -> [w338]
          shift-right: [w339] -> w326
          shift-left: _ -> [w337]
          stop <- w334 stop-if-true
          # "BB spectra"
          # "Accumulated BB spectra"
          # "Accumulated sample spectra"
          # "Sample spectra"
          # "Latest spectrum"
          n180 = case shown="True" "Pause\nacquisition" {
            tunnel: w335 -> [w355 w356]
            tunnel: [w355 w356] -> w333
            frame False {
            }
            frame True {
              n181 = while {
                stop <- w360 stop-if-true
                n182 = local read "Pause\nacquisition"() -> (w359:bool)
                n183 = Wait (ms)(milliseconds to wait=5) -> ()  [unwired: 1 out]
                n184 = local write "Acquisition status"("Paused!") -> ()
                n185 = Not(x=w359) -> (.not. x?=w360:bool)
              }
            }
          }
          n186 = Equal?(x=Control_GetSpectrum_BBnorm_AttenuateBB."Done", y=w335) -> (x = y?=w334:bool)
          n187 = case shown="\"Flip out BB\"" w333 {
            tunnel: [w361 w391 w399 w437 w492 w529 w563 w590 w612 w639 w650] -> w353
            tunnel: [w361 w392 w400 w435 w491 w540 w564 w583 w613 w638 w652] -> w352
            tunnel: w351 -> [_ w392 w400 w435 w491 w549 w564 w583 w613 w638 w652]
            tunnel: w350 -> [_ w391 w399 w437 w492 w529 w563 w591 w612 w639 w650]
            tunnel: [w367 Control_GetSpectrum_BBnorm_AttenuateBB."Flip in BB" Control_GetSpectrum_BBnorm_AttenuateBB."Attenuate alpha" w411 w476 w520 Control_GetSpectrum_BBnorm_AttenuateBB."Attenuate alpha" Control_GetSpectrum_BBnorm_AttenuateBB."Assess accumulation" w615 Control_GetSpectrum_BBnorm_AttenuateBB."Done" Control_GetSpectrum_BBnorm_AttenuateBB."Done"] -> w349
            tunnel: w348 -> [w364 w388 w402 w421 w486 w544 w562 w601 w617 w641 w654]
            tunnel: w347 -> [w363 w387 w401 w425 w493 w543 w561 w600 w618 w640 w653]
            tunnel: [w363 w382 w401 w432 w493 w534 w561 w589 w618 w640 w653] -> w346
            tunnel: [w364 w383 w402 w409 w486 w542 w562 w599 w617 w641 w654] -> w345
            tunnel: [w361 w381 w398 w436 w479 w535 w560 w593 w614 w645 w651] -> w344
            tunnel: w342 -> [_ w381 w398 w436 _ w535 w560 w593 w614 w645 w651]
            tunnel: "Toggle pause (ms)" -> [_ _ w395 _ _ _ w557 _ _ _ _]
            tunnel: [w361 w380 w397 w434 w488 w525 w559 w580 w610 w643 w648] -> w340
            tunnel: [w361 w379 w396 w433 w487 w523 w558 w581 w611 w642 w647] -> w339
            tunnel: w338 -> [_ w380 w397 w434 w488 w523 w559 w580 w610 w643 w648]
            tunnel: w337 -> [_ w379 w396 w433 w487 w524 w558 _ w611 w642 w647]
            frame "Initialize" {
              w368 = dbl[] []
              n188 = local write "Spectrum stored"(FALSE) -> ()
              n189 = local write "# Accumulated"(0) -> ()
              n190 = local read "Replicate\nalpha on\naccumulation"() -> (w365:bool)
              n191 = case shown="False" w365 {
                tunnel: [Control_GetSpectrum_BBnorm_AttenuateBB."Flip in BB" Control_GetSpectrum_BBnorm_AttenuateBB."Replicate alpha"] -> w367
                frame False {
                }
                frame True {
                  n192 = local write "Acquisition status"("Replicating alpha...") -> ()
                }
              }
              n193 = Build Array(w368, w368) -> (w361:dbl[][])
              "Sample Spectra" <- w361
              "Sample BB Spectra" <- w361
            }
            frame "Replicate alpha" {
              w385 = "replicate"
              # "Wait time for replication (s)\nExtra if we replicate for the first time"
              n194 = local write "Acquisition status"("Replicating alpha...") -> ()
              n195 = local read "# Accumulated"() -> (w375:i32)
              n196 = Add(x=w375, y="Replicate\nfrom #") -> (x+y=w377:i32)
              n197 = local read "Python alpha rep path"() -> (w386:path)
              n198 = Equal?(x=w375, y=0) -> (x = y?=w374:bool)
              n199 = case shown="False" w374 {
                tunnel: [10 15] -> w373
                frame False {
                }
                frame True {
                }
              }
              n200 = node(w388, w386, w385, w387, w385, w377, w373) -> (w383:refnum<k35>, w382:errorcluster, w384:string)  [unwired: 2 in, 2 out]
              n201 = local write "Python error: spectrum acquisition"(w382) -> ()
              n202 = local write "Latest alpha cmd"(w384) -> ()
              n203 = local write "Attenuation factor"(1) -> ()
            }
            frame "Flip in BB" {
              n204 = flat-sequence {
                tunnel: w395 -> [w405]
                frame #0 {
                  n205 = local write "Acquisition status"("Toggling to bright beam...") -> ()
                }
                frame #1 {
                  n206 = local write "Toggle position"(1) -> ()
                  n207 = call "NewportFlipper.vi"("Settle time (ms)"=w405, "Up/Down"=TRUE) -> ()  [unwired: 10 in]
                }
                frame #2 {
                  n208 = local write "Acquisition status"("Acquiring bright beam spectrum...") -> ()
                }
              }
            }
            frame "Attenuate alpha" {
              w431 = "set_pump"
              # "If replicating alpha on accumulation,\nuse table of attenuation"
              n209 = local read "Toggle position"() -> (w416:i32)
              n210 = local read "Replicate\nalpha on\naccumulation"() -> (w422:bool)
              n211 = local read "Replicator wavelengths loaded"() -> (w427:bool)
              n212 = Equal?(x=w416, y=1) -> (x = y?=w417:bool)
              n213 = case shown="True" w417 {
                tunnel: ["Sample power (%)" "BB power (%)"] -> w414
                tunnel: ["Sample atten.\npowers (%)" "BB attenuation\npowers (%)"] -> w413
                frame False {
                }
                frame True {
                }
              }
              n214 = flat-sequence {
                tunnel: w421 -> [w464]
                tunnel: [w464] -> w420
                frame #0 {
                  n215 = local write "Acquisition status"("Attenuating alpha for BB spectrum") -> ()
                }
              }
              n216 = And(x=w422, y=w427) -> (x .and. y?=w428:bool)
              n217 = local read "Python alpha rep path"() -> (w426:path)
              n218 = case shown="True" w428 {
                tunnel: [w447 w452] -> w412
                tunnel: w420 -> [w449 w459]
                tunnel: w426 -> [_ w458]
                tunnel: w425 -> [w448 w456]
                tunnel: [w449 w455] -> w424
                tunnel: [w448 w454] -> w423
                tunnel: w414 -> [w447 _]
                tunnel: w413 -> [_ w451]
                frame False {
                }
                frame True {
                  n219 = local read "Replication wavelengths"() -> (w461:dbl[])
                  n220 = local read "# Accumulated"() -> (w462:i32)
                  n221 = local read "Replicate\nfrom #"() -> (w463:i8)
                  n222 = Add(x=w462, y=w463) -> (x+y=w460:i32)
                  n223 = Index Array(array=w461, index=w460) -> (element=w450:dbl)
                  "Replicated wavelength (nm)" <- w450
                  n224 = node(w459, w458, "get_pump_at_replication_wavelength", w456, w450, w450, "Attenuation\nenergies (cm-1)", w451) -> (w455:refnum<k35>, w454:errorcluster, w452:dbl)  [unwired: 3 in, 2 out]
                }
              }
              n225 = Divide(x=w412, y=100) -> (x/y=w418:dbl)
              n226 = node(w424, w426, w431, w423, w431, w412) -> (w419:refnum<k35>, w432:errorcluster, w430:string)  [unwired: 1 in, 2 out]
              n227 = local write "Latest alpha cmd"(w430) -> ()
              n228 = flat-sequence {
                tunnel: w419 -> [w446]
                tunnel: [w446] -> w410
                tunnel: w418 -> [w445]
                frame #0 {
                  "Attenuation factor" <- w445
                }
              }
              n229 = flat-sequence {
                tunnel: [Control_GetSpectrum_BBnorm_AttenuateBB."Get Spectrum"] -> w411
                tunnel: w410 -> [w439]
                tunnel: [w439] -> w409
                frame #0 {
                  n230 = local write "Acquisition status"("Acquiring spectrum...") -> ()
                }
              }
            }
            frame "Get Spectrum" {
              n231 = control-ref of="% averaged"() -> (w484:refnum<vi>)
              n232 = control-ref of="Acquisition cycle"() -> (w483:refnum<vi>)
              n233 = control-ref of="Cancel\nacquisition"() -> (w478:refnum<vi>)
              n234 = local read "Toggle position"() -> (w490:i32)
              n235 = control-ref of="Binned interferogram"() -> (w485:refnum<vi>)
              n236 = Equal?(x=w490, y=1) -> (x = y?=w468:bool)
              n237 = case shown="True" w468 {
                tunnel: ["Sample: physical channels (inputV, ScanDelay X)" "Bright beam: physical channels (inputV, ScanDelay X)"] -> w473
                tunnel: [w500 w502] -> w472
                frame False {
                  n238 = local read "Sample: alignment delay"() -> (w500:i32)
                }
                frame True {
                  n239 = local read "Bright beam: alignment delay"() -> (w502:i32)
                }
              }
              n240 = And(x="Optimize\ninterferogram\nalignment", y="Update alignment") -> (x .and. y?=w469:bool)
              n241 = case shown="True" w468 {
                tunnel: ["Cyc. / intfg.\n(sample)" "Cyc. per intfg. (BB)"] -> w467
                frame False {
                }
                frame True {
                }
              }
              n242 = call "ScanDelay_FTIR_GetSpectrum_Aligning.vi"("Cancel? External"=w478, "% averaged (external)"=w484, "Binned interferogram (external)"=w485, "Python refnum in"=w486, "Optimize\ninterferogram\ndelay"="Optimize\ninterferogram\nalignment", "Acquisition cycle (external)"=w483, "Gain"=1.0, "Displacement\n calibration  factor"="Delay calibratior\nfactor (ps/V)", "Channels to read (input V, ScanDelay)"=w473, "Acquisitions per interferogram"=w467, "Time per\nacquisition (s)"="Time per\nacquisition (s)", "Sampling rate"="Sampling rate", "Delay estimation (pts)"=w472) -> ("Output spectrum"=w479:dbl[][], "Best delay"=w474:i32)  [unwired: 1 in]
              n243 = case shown="True" w469 {
                tunnel: w474 -> [_ w497]
                tunnel: w468 -> [_ w496]
                frame False {
                }
                frame True {
                  # "Update our optimal delay only if we are actively optimizing"
                  n244 = case shown="True" w496 {
                    tunnel: w497 -> [w498 w499]
                    frame False {
                      n245 = local write "Sample: alignment delay"(w498) -> ()
                    }
                    frame True {
                      n246 = local write "Bright beam: alignment delay"(w499) -> ()
                    }
                  }
                }
              }
              n247 = case shown="True" w468 {
                tunnel: [Control_GetSpectrum_BBnorm_AttenuateBB."Accumulate sample spectrum" Control_GetSpectrum_BBnorm_AttenuateBB."Accumulate BB spectrum"] -> w477
                tunnel: w479 -> [_ _]
                tunnel: [w506 w511] -> w475
                frame False {
                  n248 = local read "Cancel\nacquisition"() -> (w507:bool)
                  n249 = local read "Halt program"() -> (w508:bool)
                  n250 = Or(x=w507, y=w508) -> (x .or. y?=w506:bool)
                  n251 = local write "Acquisition status"("Accumulating sample spectrum...") -> ()
                }
                frame True {
                  n252 = local read "Cancel\nacquisition"() -> (w513:bool)
                  n253 = local read "Halt program"() -> (w512:bool)
                  n254 = Or(x=w513, y=w512) -> (x .or. y?=w511:bool)
                  n255 = local write "Acquisition status"("Accumulating bright beam spectrum...") -> ()
                }
              }
              n256 = case shown="True" w475 {
                tunnel: w477 -> [w504 _]
                tunnel: [w504 Control_GetSpectrum_BBnorm_AttenuateBB."Done"] -> w476
                frame False {
                }
                frame True {
                }
              }
            }
            frame "Accumulate BB spectrum" {
              n257 = local read "# Accumulated"() -> (w548:i32)
              n258 = Equal?(x=w548, y=0) -> (x = y?=w546:bool)
              n259 = case shown="False" w546 {
                tunnel: w535 -> [w554 w556]
                tunnel: w549 -> [w555 _]
                tunnel: [w553 w556] -> w540
                frame False {
                  n260 = Build Array (concatenate)(w555, w554) -> (w553:dbl[][])
                }
                frame True {
                }
              }
              n261 = local read "Apply spectral\nenvelope"() -> (w522:bool)
              n262 = local read "Python scandelay path"() -> (w541:path)
              n263 = local read "Envelope width"() -> (w521:dbl)
              n264 = node(w544, w541, "accumulate_spectra", w543, w540, w540, w522, w521) -> (w542:refnum<k35>, w534:errorcluster, w525:dbl[][])  [unwired: 3 in, 2 out]
              n265 = Index Array(array=w525, index (row) #1=0, index (row) #2=1) -> (element #1=w537:dbl[], element #2=w536:dbl[])  [unwired: 2 in]
              n266 = Index Array(array=w524, index (row) #1=0, index (row) #2=1) -> (element #1=w531:dbl[], element #2=w530:dbl[])  [unwired: 2 in]
              n267 = Bundle("Output spectrum"=w537, "Output spectrum"=w536) -> (w527:T1)  [unwired: 1 in]
              n268 = Bundle("Output spectrum"=w531, "Output spectrum"=w530) -> (w528:T1)  [unwired: 1 in]
              n269 = local write "Python error: spectrum acquisition"(w534) -> ()
              n270 = Build Array(w528, w527) -> (→"Accumulated spectrum (amplitude)":T3)
              n271 = Not(x="Flip anyway") -> (.not. x?=w518:bool)
              n272 = And(x="Acquire only\nBB 100% curve", y=w518) -> (x .and. y?=w517:bool)
              n273 = case shown="False" w517 {
                tunnel: [Control_GetSpectrum_BBnorm_AttenuateBB."Flip out BB" Control_GetSpectrum_BBnorm_AttenuateBB."Attenuate alpha"] -> w520
                frame False {
                }
                frame True {
                  n274 = local write "Toggle position"(2) -> ()
                }
              }
            }
            frame "Flip out BB" {
              n275 = flat-sequence {
                tunnel: w557 -> [w568]
                tunnel: w557 -> [w574]
                frame #0 {
                  n276 = local write "Acquisition status"("Toggling to sample beam ...") -> ()
                }
                frame #1 {
                  n277 = local write "Toggle position"(2) -> ()
                  n278 = call "NewportFlipper.vi"("Settle time (ms)"=w568, "Up/Down"=FALSE) -> ()  [unwired: 10 in]
                }
                frame #2 {
                  w570 = "Returning to bright beam..."
                  n279 = local read "Acquire only\nBB 100% curve"() -> (w573:bool)
                  n280 = local read "Flip anyway"() -> (w572:bool)
                  n281 = local write "Acquisition status"(w570) -> ()
                  n282 = And(x=w573, y=w572) -> (x .and. y?=w571:bool)
                  n283 = case shown="True" w571 {
                    tunnel: w574 -> [_ w575]
                    tunnel: w570 -> [_ _]
                    frame False {
                    }
                    frame True {
                      n284 = call "NewportFlipper.vi"("Settle time (ms)"=w575, "Up/Down"=TRUE) -> ()  [unwired: 10 in]
                    }
                  }
                }
                frame #3 {
                  n285 = local write "Acquisition status"("Acquiring sample beam spectrum...") -> ()
                }
              }
            }
            frame "Accumulate sample spectrum" {
              (unwired) 0
              n286 = local read "# Accumulated"() -> (w605:i32)
              n287 = Equal?(x=w605, y=0) -> (x = y?=w603:bool)
              n288 = case shown="True" w603 {
                tunnel: w593 -> [w607 w609]
                tunnel: w591 -> [w608 _]
                tunnel: [w606 w609] -> w590
                frame False {
                  n289 = Build Array (concatenate)(w608, w607) -> (w606:dbl[][])
                }
                frame True {
                }
              }
              n290 = local read "Apply spectral\nenvelope"() -> (w579:bool)
              n291 = local read "Python scandelay path"() -> (w598:path)
              n292 = local read "Envelope width"() -> (w578:dbl)
              n293 = node(w601, w598, "accumulate_spectra", w600, w590, w590, w579, w578) -> (w599:refnum<k35>, w589:errorcluster, w581:dbl[][])  [unwired: 3 in, 2 out]
              n294 = local write "Python error: spectrum acquisition"(w589) -> ()
              n295 = Index Array(array=w581, index (row) #1=0, index (row) #2=1) -> (element #1=w595:dbl[], element #2=w594:dbl[])  [unwired: 2 in]
              n296 = Index Array(array=w580, index (row) #2=1) -> (element #1=w586:dbl[], element #2=w585:dbl[])  [unwired: 3 in]
              n297 = Bundle("Output spectrum"=w595, "Output spectrum"=w594) -> (w588:T1)  [unwired: 1 in]
              n298 = Bundle("Output spectrum"=w586, "Output spectrum"=w585) -> (w584:T1)  [unwired: 1 in]
              n299 = Build Array(w588, w584) -> (w582:T3)
              n300 = property on="Accumulated spectrum (amplitude)" class="XYGraph (strict)"("Value"=w582) -> ()  [unwired: 2 in, 2 out]
            }
            frame "Assess accumulation" {
              n301 = flat-sequence {
                tunnel: [w623] -> w616
                tunnel: w613 -> [w622]
                tunnel: w612 -> [w621]
                tunnel: w611 -> [w619]
                tunnel: w610 -> [w620]
                tunnel: w616 -> [w625]
                tunnel: [w629] -> w615
                frame #0 {
                  n302 = local read "# Accumulated"() -> (w624:i32)
                  n303 = local write "Accumulated sample spectrum"(w619) -> ()
                  n304 = Increment(x=w624) -> (x+1=w623:i32)
                  n305 = local write "Accumulated sample BB spectrum"(w620) -> ()
                  n306 = local write "Sample Spectra"(w621) -> ()
                  n307 = local write "Sample BB Spectra"(w622) -> ()
                  n308 = local write "# Accumulated"(w623) -> ()
                }
                frame #1 {
                  n309 = local read "Accumulate to #"() -> (w626:i32)
                  n310 = property on="BB-reference spectrum" class="Bool (strict)"("Val(Sgnl)"=TRUE) -> ()  [unwired: 2 in, 2 out]
                  n311 = Less Or Equal?(x=w626, y=w625) -> (x <= y?=w627:bool)
                  n312 = case shown="False" w627 {
                    tunnel: [w630 Control_GetSpectrum_BBnorm_AttenuateBB."Finalize"] -> w629
                    frame False {
                      n313 = local read "Replicate\nalpha on\naccumulation"() -> (w631:bool)
                      n314 = case shown="True" w631 {
                        tunnel: [Control_GetSpectrum_BBnorm_AttenuateBB."Flip in BB" Control_GetSpectrum_BBnorm_AttenuateBB."Replicate alpha"] -> w630
                        frame False {
                          n315 = local write "Acquisition status"("Toggling to bright beam") -> ()
                        }
                        frame True {
                          n316 = local write "Acquisition status"("Replicating alpha...") -> ()
                        }
                      }
                    }
                    frame True {
                    }
                  }
                }
              }
            }
            frame "Finalize" {
              n317 = local write "Spectrum stored"(TRUE) -> ()
            }
            frame "Done" {
              w646 = FALSE
              n318 = local write "Acquire spectrum"(w646) -> ()
              n319 = local write "Cancel\nacquisition"(w646) -> ()
            }
          }
          n320 = Wait (ms)(milliseconds to wait=5) -> ()  [unwired: 1 out]
        }
      }
      event Timeout {
        n321 = event-data() -> ()  [unwired: 1 in, 3 out]
        n322 = Wait (ms)(milliseconds to wait=w657) -> ()  [unwired: 1 out]
      }
    }
    n323 = Wait (ms)(milliseconds to wait=5) -> ()  [unwired: 1 out]
    n324 = local read "Halt program"() -> (w325:bool)
    "Acquisition status" <- "Ready to acquire spectrum"
  }
  n325 = Close Python Session(session in=w13, error in=w12) -> (11:w9:errorcluster)
  n326 = local write "Python error: activity loop"(w9) -> ()
  n327 = Close Python Session(session in=w3, error in=w2) -> ()  [unwired: 1 out]
